vi "Text control 2 v5.9.vi"() -> ()   [LabVIEW 2016]
panel:
  in  "Tab Control":enum32{"Main", "Other parameters"}(tab)
  out "Line running":i32
  out "Total lines":i32
  out "Path":path=path "C:/users/rlp38/09Apr2009LTtesting/test2.txt"
  out "I vs Vg":cluster{"Y data in":dbl[], "X data in":dbl[]}[](graph)
  out "Is max":dbl format="%.2e"
  out "Id max":dbl format="%.2e"
  out "Ig max":dbl format="%.2e"
  out "Imax vs time":cluster{"Y data in":dbl[], "X data in":dbl[]}[](graph)
  out "Imin vs time":cluster{"Y data in":dbl[], "X data in":dbl[]}[](graph)
  out "I vs Vd":cluster{"Y data in":dbl[], "X data in":dbl[]}[](graph)
  in  "Script":string="#pulsedstressV d 0.03 20 0 0.5 0.0827 5\n#\n#itime m\n#gaterangemode a\n#drainrangemode a\n#pulsed on 0.05 0 0.02\n#transfer d -10 40 1 5 40 35\n#transfer d -10 40 1 5 40 35\n#transfer d -10 40 1 5 40 35\n#output d 0 40 20 0 40 1\n#\n#\n#sample 1 0.008 221 6 0.003\n#samplei 400e-6 200 6 0.002 0.1\n#vsu2pulse -10 4\n#\n#stressV 0.016 0.03 2e-4 0.1e-3 11\n#stressI 220e-7 0.08 15\n#transfer s -1 1 0.5 -0.005 0.005 0.005\n#output s 0 0 0 -0.008 0.008 0.002"
  out "Command running:":string
  out "Serial port data":string
  out "Elapsed Time":dbl caption="Elapsed Time (s)"
  in  "Units (label only)":u16(ring)=1 items=["Seconds", "Minutes", "Hours"]
  in  "Time Offset":dbl caption="Set Start Time (s)"
  in  "Reset":bool
  in  "Auto Reset":bool
  in  "integration time":u32(slide) max=2 step=1 scale=0.0..2.0
  out "Is on":dbl format="%.2e"
  out "Id on":dbl format="%.2e"
  out "Ig on":dbl format="%.2e"
  out "Ion vs time":cluster{"Y data in":dbl[], "X data in":dbl[]}[](graph)
  out "Ioff vs time":cluster{"Y data in":dbl[], "X data in":dbl[]}[](graph)
  out "Ig min":dbl format="%.2e"
  out "Id min":dbl format="%.2e"
  out "Is min":dbl format="%.2e"
  out "Is off":dbl format="%.2e"
  out "Id off":dbl format="%.2e"
  out "Ig off":dbl format="%.2e"
  in  "Integration time (long)":dbl=0.32 min=0.04 max=2.0 step=0.02 format="%.2f"
  in  "Integration time (short)":dbl=0.0019 min=8e-05 max=0.0019 step=8e-05 format="%^.0e"
  in  "Drain: Compliance":dbl=0.001 format="%.8f"
  in  "Gate: Compliance":dbl=0.001 format="%.8f"
  in  "Interrupt run":bool
  in  "Standby":T1
  in  "Full Reset":bool
  in  "SMU4":cluster{"on/off":bool, "Voltage":dbl} {"Voltage" min=-100.0 max=100.0 format="%.2f"}
  in  "Gate Range\nmode":u16(ring) items=["Auto", "Limited", "Fixed"]
  in  "Gate Range":u8(slide)=6 max=11 scale=0.0..11.0
  in  "Source/Drain\nRange mode":u16(ring) items=["Auto", "Limited", "Fixed"]
  in  "Source/Drain Range":u8(slide)=6 max=11 scale=0.0..11.0
  in  "Panel Controls":T2={"Emergency Stop"=refnum, "TransGraph Max"=1e-05, "Text/Graph (text=false)"=TRUE} {"TransGraph Max" format="%.2e"}
  in  "Panel Controls 2":T3={"Emergency Stop"=refnum, "TransGraph Max"=1e-05, "Text/Graph (text=false)"=TRUE, "TransGraph Min"=1e-11} {"TransGraph Min" format="%.2e"; "TransGraph Max" format="%.2e"}
  out "error out":errorcluster
  in  "Delay before read (ms)":u32=1000
  in  "byte count":u32=64
  in  "Serial End Mode for Reads":u16(ring)=2 items=["None", "LastBit", "TermChar"]
  in  "Timeout (ms)":u32=10000
  in  "Enable Termination\nChar (T)":bool=TRUE
  in  "Termination char\n(0xA = '\\n' = LF)\n(0xD = '\\r' = CR)":u8=13 format="%.0x"
  in  "flow control":u16(ring) items=["None"=0, "XON/XOFF"=1, "RTS/CTS"=2, "DTR/DSR"=4]
  in  "stop bits":u16(ring)=10 items=["1.0"=10, "1.5"=15, "2.0"=20]
  in  "parity":u16(ring) items=["None", "Odd", "Even", "Mark", "Space"]
  in  "data bits":u16=8 min=5 max=8 step=1
  in  "VISA resource name":refnum<visa-resource-name>="COM6"
  in  "baud rate":u32=9600
  out "Timings Indicator":T4
  in  "Timings (overwritten by the Front Panel)":T5={"integration time"=0, "Short/Long integration time"=0.00064, "hold time (sec)"=0.0, "delay time (sec)"=0.0, "Step Time (0 disables)"=0.0, "sweep method"=0, "Pulse period"=0.005, "Base voltage"=0.0, "Pulse width"=0.0005} {"Pulse width" min=0.0005 max=0.1 step=0.0001 format="%.4f"; "Base voltage" format="%^.4e"; "Pulse period" min=0.005 max=1.0 step=0.0001 format="%.4f"; "sweep method" items=["Continuous", "Pulsed"]; "Step Time (0 disables)" format="%.2f"; "delay time (sec)" format="%.4f"; "hold time (sec)" format="%.4f"; "Short/Long integration time" format="%^.0e"; "integration time" scale=0.0..2.0}
  in  "Gate":T6={"Gate Start"=0.0, "Gate Stop"=2.0, "Gate Step (linear only)"=1.0, "Gate Compliance"=0.0001, "Gate PComp"=0.0, "Range mode"=0, "Range"=6} {"Range" max=11 scale=0.0..11.0; "Range mode" items=["Auto", "Limited", "Fixed"]; "Gate PComp" format="%^.2e"; "Gate Compliance" format="%^.2e"; "Gate Step (linear only)" format="%^.4e"; "Gate Stop" format="%^.4e"; "Gate Start" format="%^.4e"}
  in  "Drain 2":T7={"Drain Start"=0.0, "Drain Stop"=2.0, "Drain Compliance"=0.0001, "Drain Step"=1.0, "Drain PComp"=0.0, "Range mode"=0, "Range"=6} {"Range" max=11 scale=0.0..11.0; "Range mode" items=["Auto", "Limited", "Fixed"]; "Drain PComp" format="%^.2e"; "Drain Step" format="%^.4e"; "Drain Compliance" format="%^.2e"; "Drain Stop" format="%^.4e"; "Drain Start" format="%^.4e"}
  # "Time"
  # "Syntax:\nitime [s|m|l] time(sec): [s|m|l] determines the integration time setting (small|medium|long) and time sets the value.\nNOTE: The value of the integration time has to be within the range allowed by its category (s|m|l), otherwise, the closest value will be used. (e.g. if the category is set to short but the time value is very long, the actual value used will be the maximum short integration time.\nIntegration times:\n    Short: Default: 640 us. Range: 8E-5 - 1.92E-3 seconds.\n    Medium: Fixed at 1 NPL cycle (0.02 seconds).\n    Long: Default: 16 NPL cycles (0.32 seconds). Range: 2-100 NPL cycles (0.04 seconds - 2 seconds).\ngaterangemode [a|l|f]\ndrainrangemode [a|l|f]\npulsed [on|off] PulsePeriod(sec) PulseBaseVoltage PulseONWidth(sec)\nstandby [on l off]\nwait NumMilliseconds\nwait-min NumMinutes\n# texthere = comment\ntransfer [s|d] VgStart VgStop VgStep VdStart VdStop VdStep\noutput [s|d] VgStart VgStop VgStep VdStart VdStop VdStep\nsample Vg Vd NumSamples Time(s) SampleInterval(s)\nsamplei Idg NumSamples Time(s) SampleInterval(s) VDGcompliance\n100 samples is approximately 13 seconds with medium integration\n# if in doubt use SampleInterval(s) = 0.004\nstressV VG VD IGcompliance IDcompliance Duration(sec)\nstressI IDG VDGcompliance Duration(sec)\nvsu2pulse Bias Duration(s)\npulsedstressV [s|d] VEstop VgON VgOFF Period(s) PulseONwidth(s) Vd\nsample-fpp Vg Vd NumSamples Time\nresample-fpp Vg Vd\ntransfer-fpp [s|d] VgStart VgStop VgStep VdStart VdStop VdStep\noutput-fpp [s|d] VgStart VgStop VgStep VdStart VdStop VdStep\nserial SerialPortCommand"
  # "1\n2\n3\n4\n5\n6\n7\n8\n9\n10\n11\n12\n13\n14\n15\n16\n17\n18\n19\n20"
  # "Serial port settings"
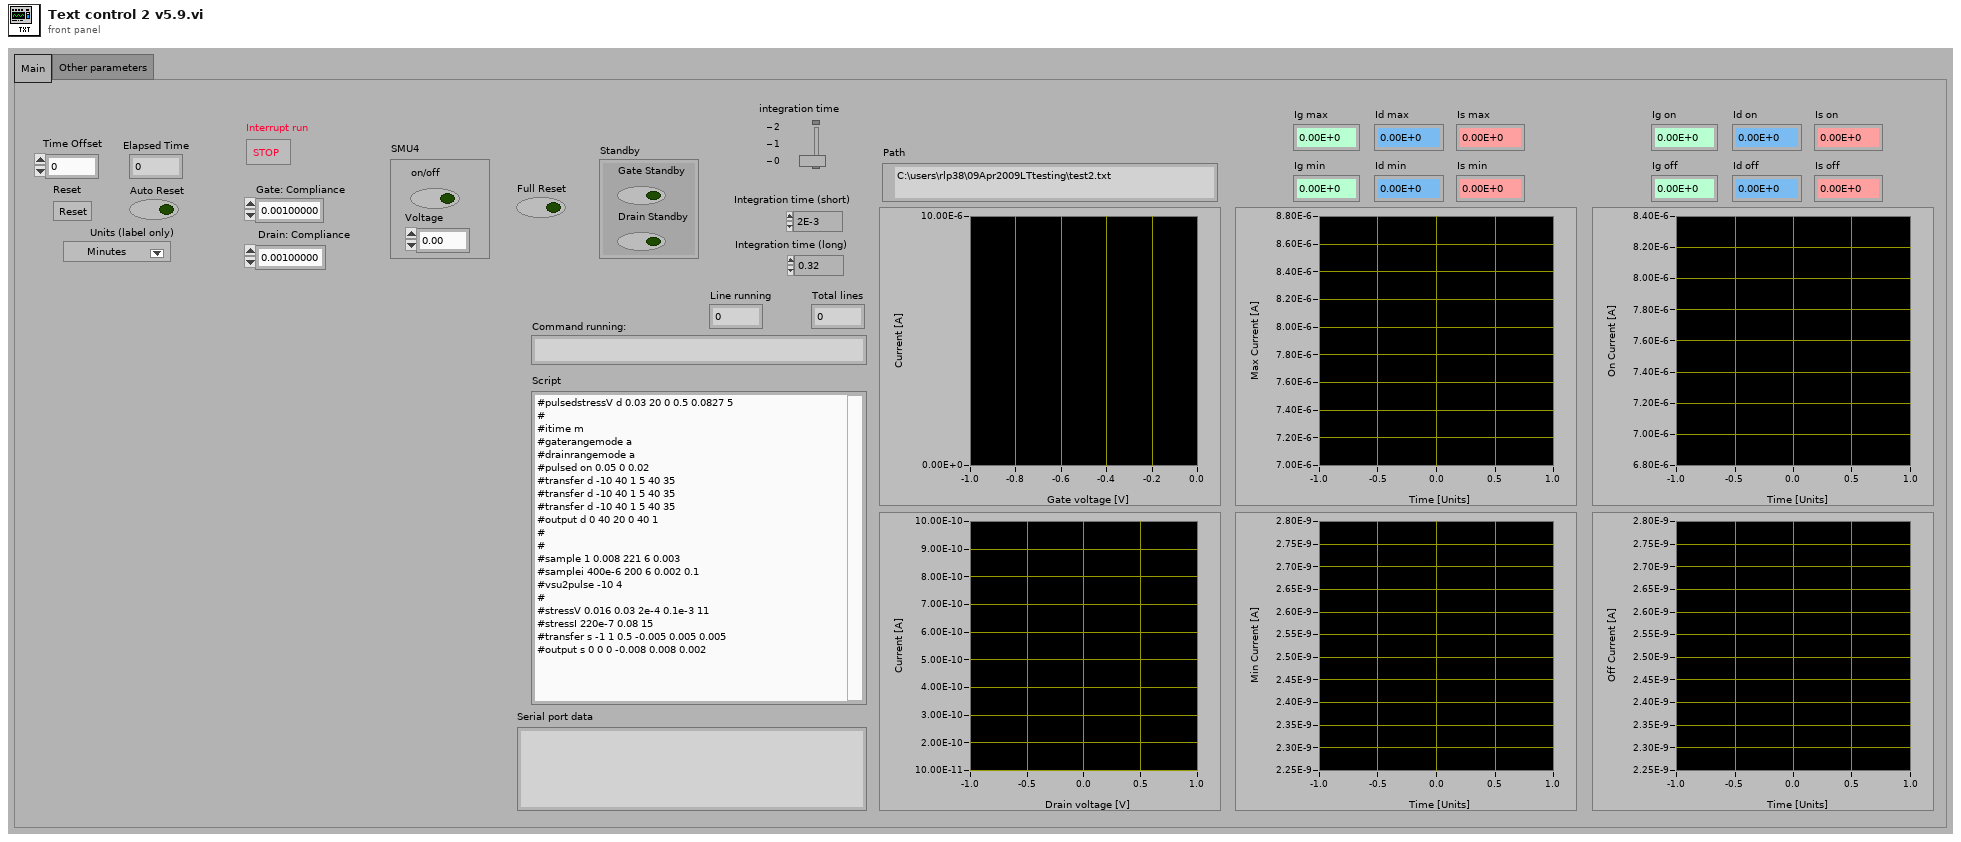
[diagram p1: front panel]
types:
  T1 = cluster{"Gate Standby":bool, "Drain Standby":bool}
  T2 = cluster{"Emergency Stop":refnum<vi>, "TransGraph Max":dbl, "Text/Graph (text=false)":bool}
  T3 = cluster{"Emergency Stop":refnum<vi>, "TransGraph Max":dbl, "Text/Graph (text=false)":bool, "TransGraph Min":dbl}
  T4 = cluster{"integration time (0:s, 1:m, 2:l)":u32, "Short/Long integration time":dbl, "hold time (sec)":dbl, "delay time (sec)":dbl, "Step Time (0 disables)":dbl, "sweep method":u16, "Pulse period":dbl, "Base voltage":dbl, "Pulse width":dbl}
  T5 = cluster{"integration time":u32, "Short/Long integration time":dbl, "hold time (sec)":dbl, "delay time (sec)":dbl, "Step Time (0 disables)":dbl, "sweep method":u16, "Pulse period":dbl, "Base voltage":dbl, "Pulse width":dbl}
  T6 = cluster{"Gate Start":dbl, "Gate Stop":dbl, "Gate Step (linear only)":dbl, "Gate Compliance":dbl, "Gate PComp":dbl, "Range mode":u16, "Range":u8}
  T7 = cluster{"Drain Start":dbl, "Drain Stop":dbl, "Drain Compliance":dbl, "Drain Step":dbl, "Drain PComp":dbl, "Range mode":u16, "Range":u8}
  T8 = enum16{"open", "replace", "create", "open or create", "replace or create", "replace or create with confirmation"}
  T9 = cluster{"V2 Start":dbl, "V2 Step":dbl, "Number of points":i32}
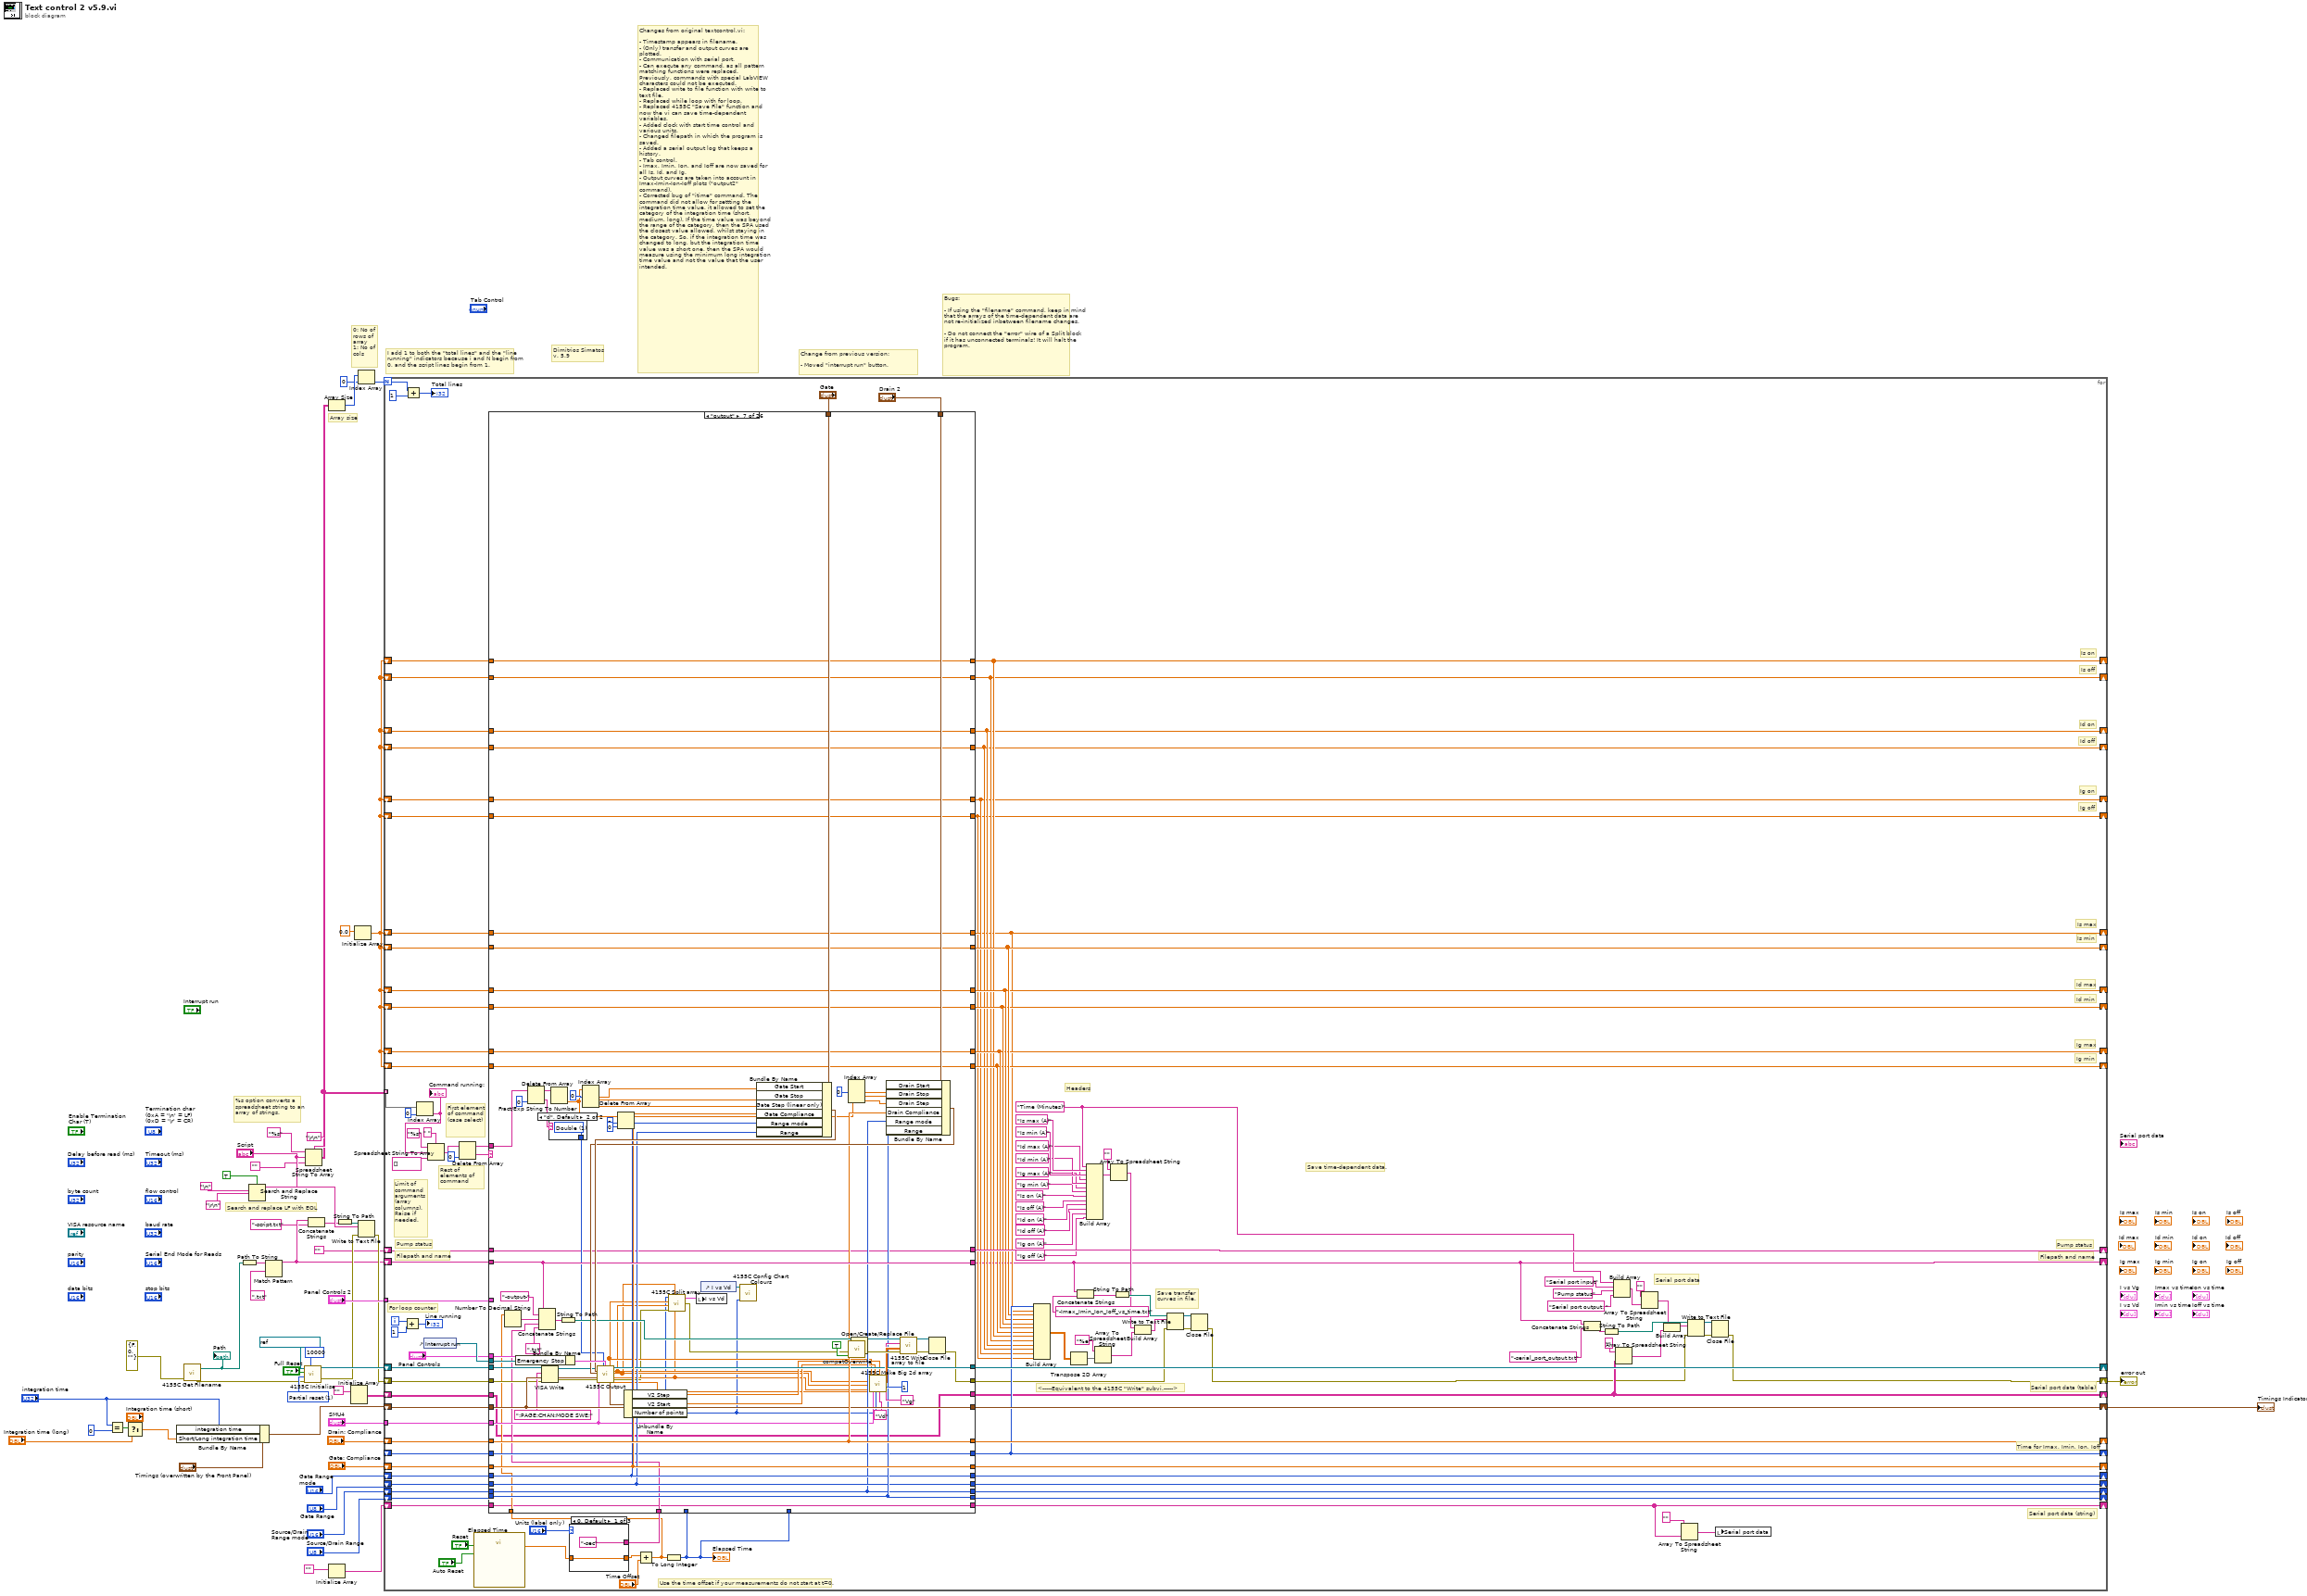
[diagram p0: block diagram]
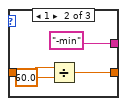
[diagram p2: hidden frame]
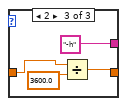
[diagram p3: hidden frame]
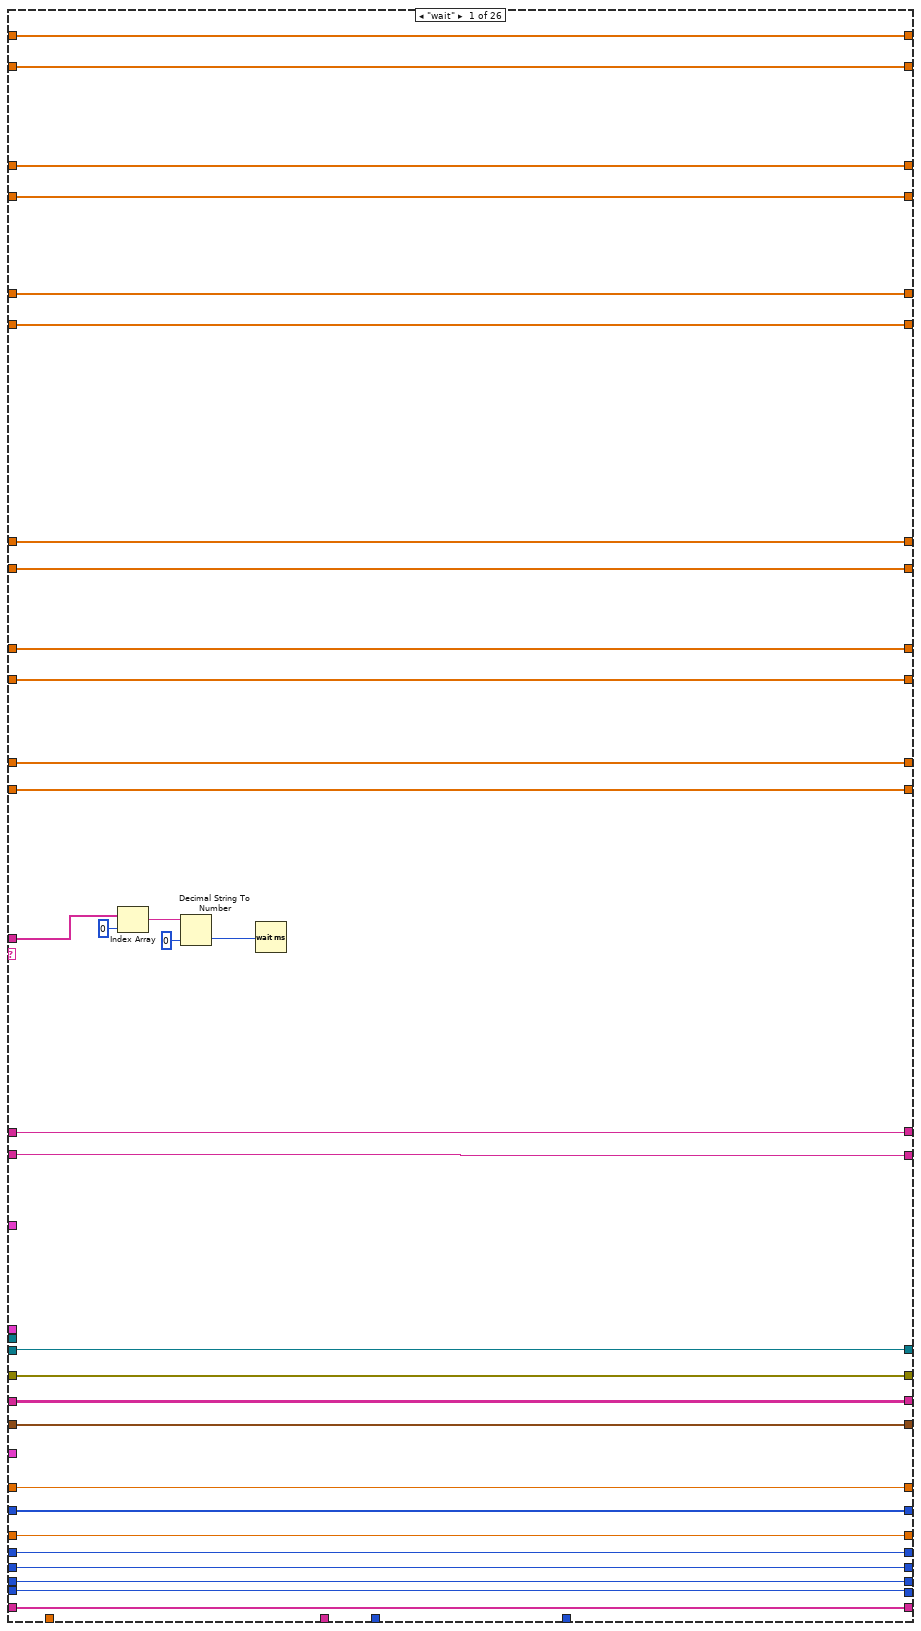
[diagram p4: hidden frame]
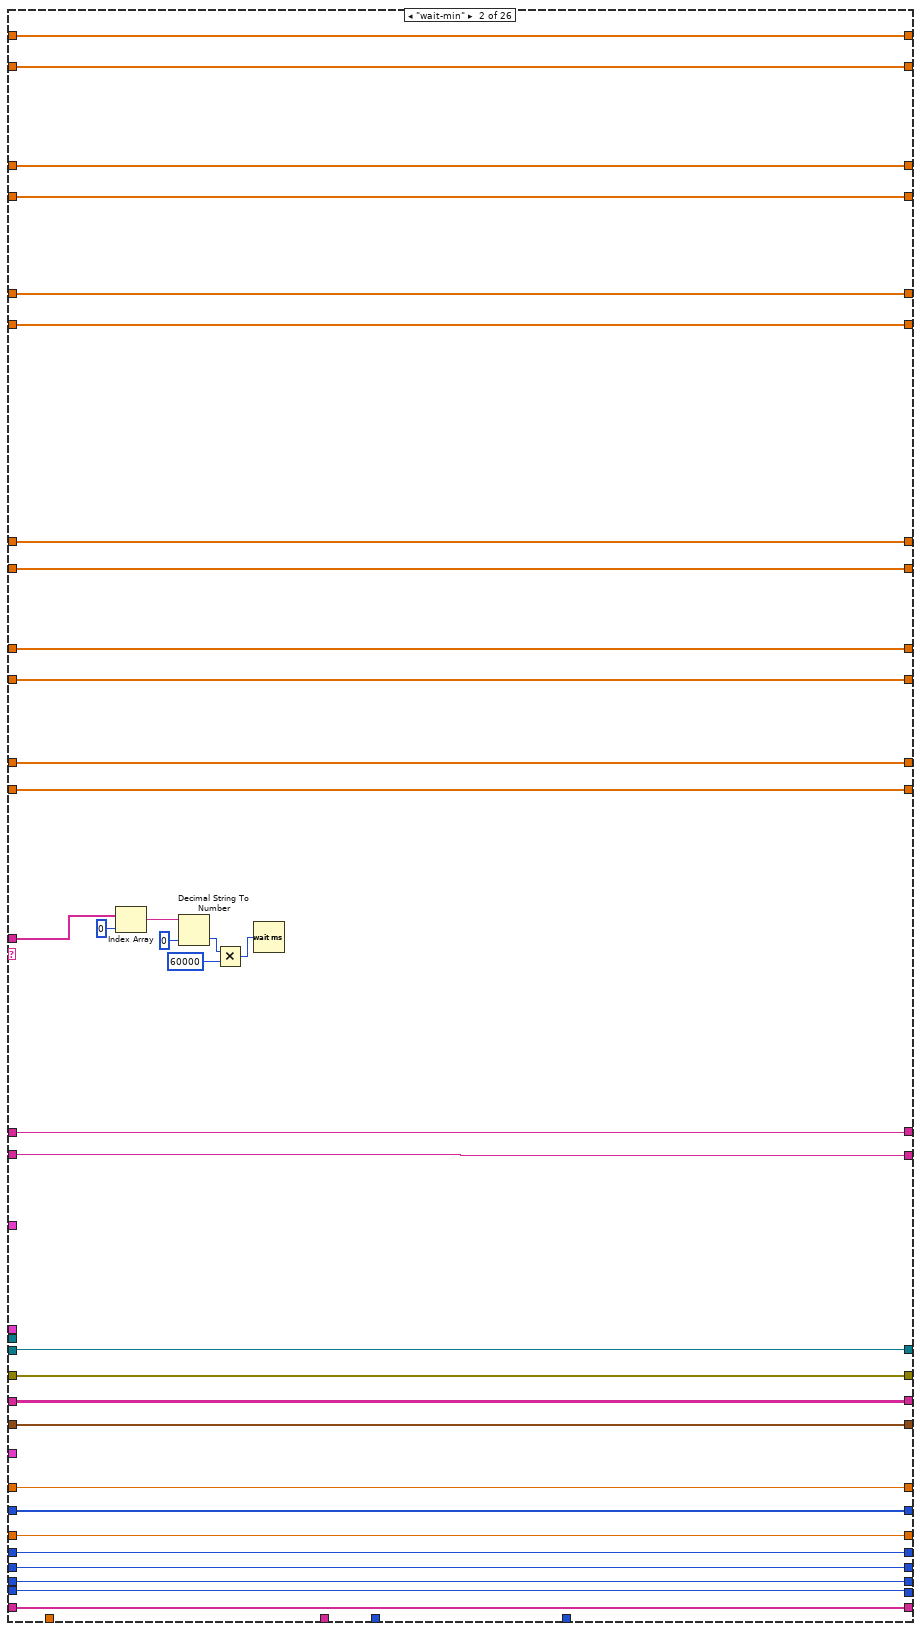
[diagram p5: hidden frame]
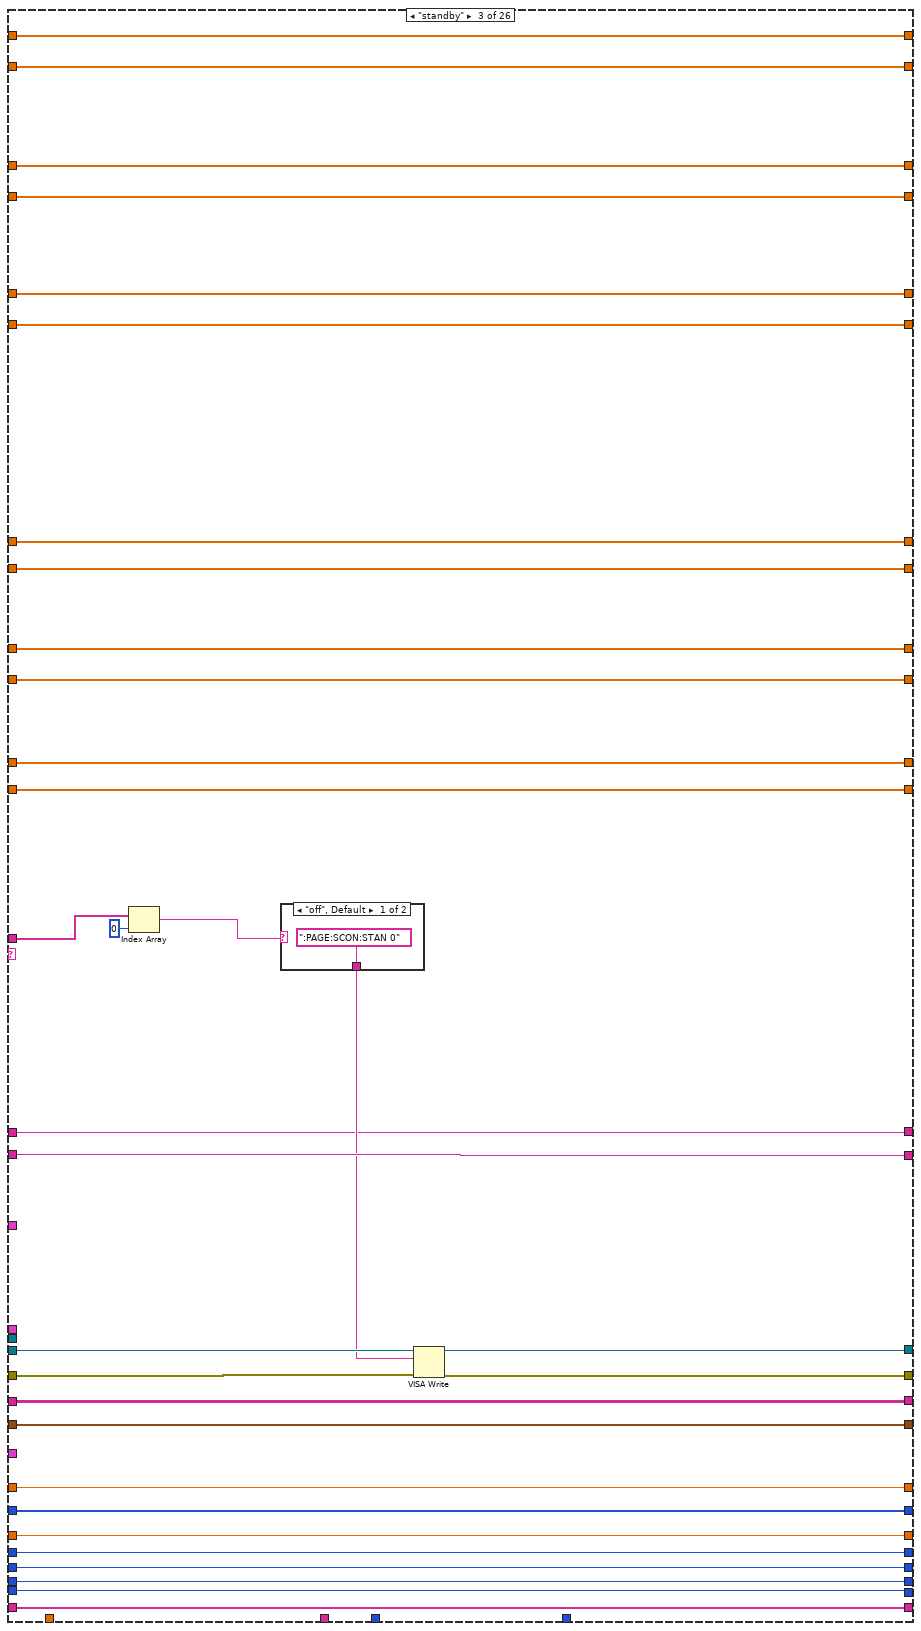
[diagram p6: hidden frame]
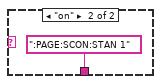
[diagram p7: hidden frame]
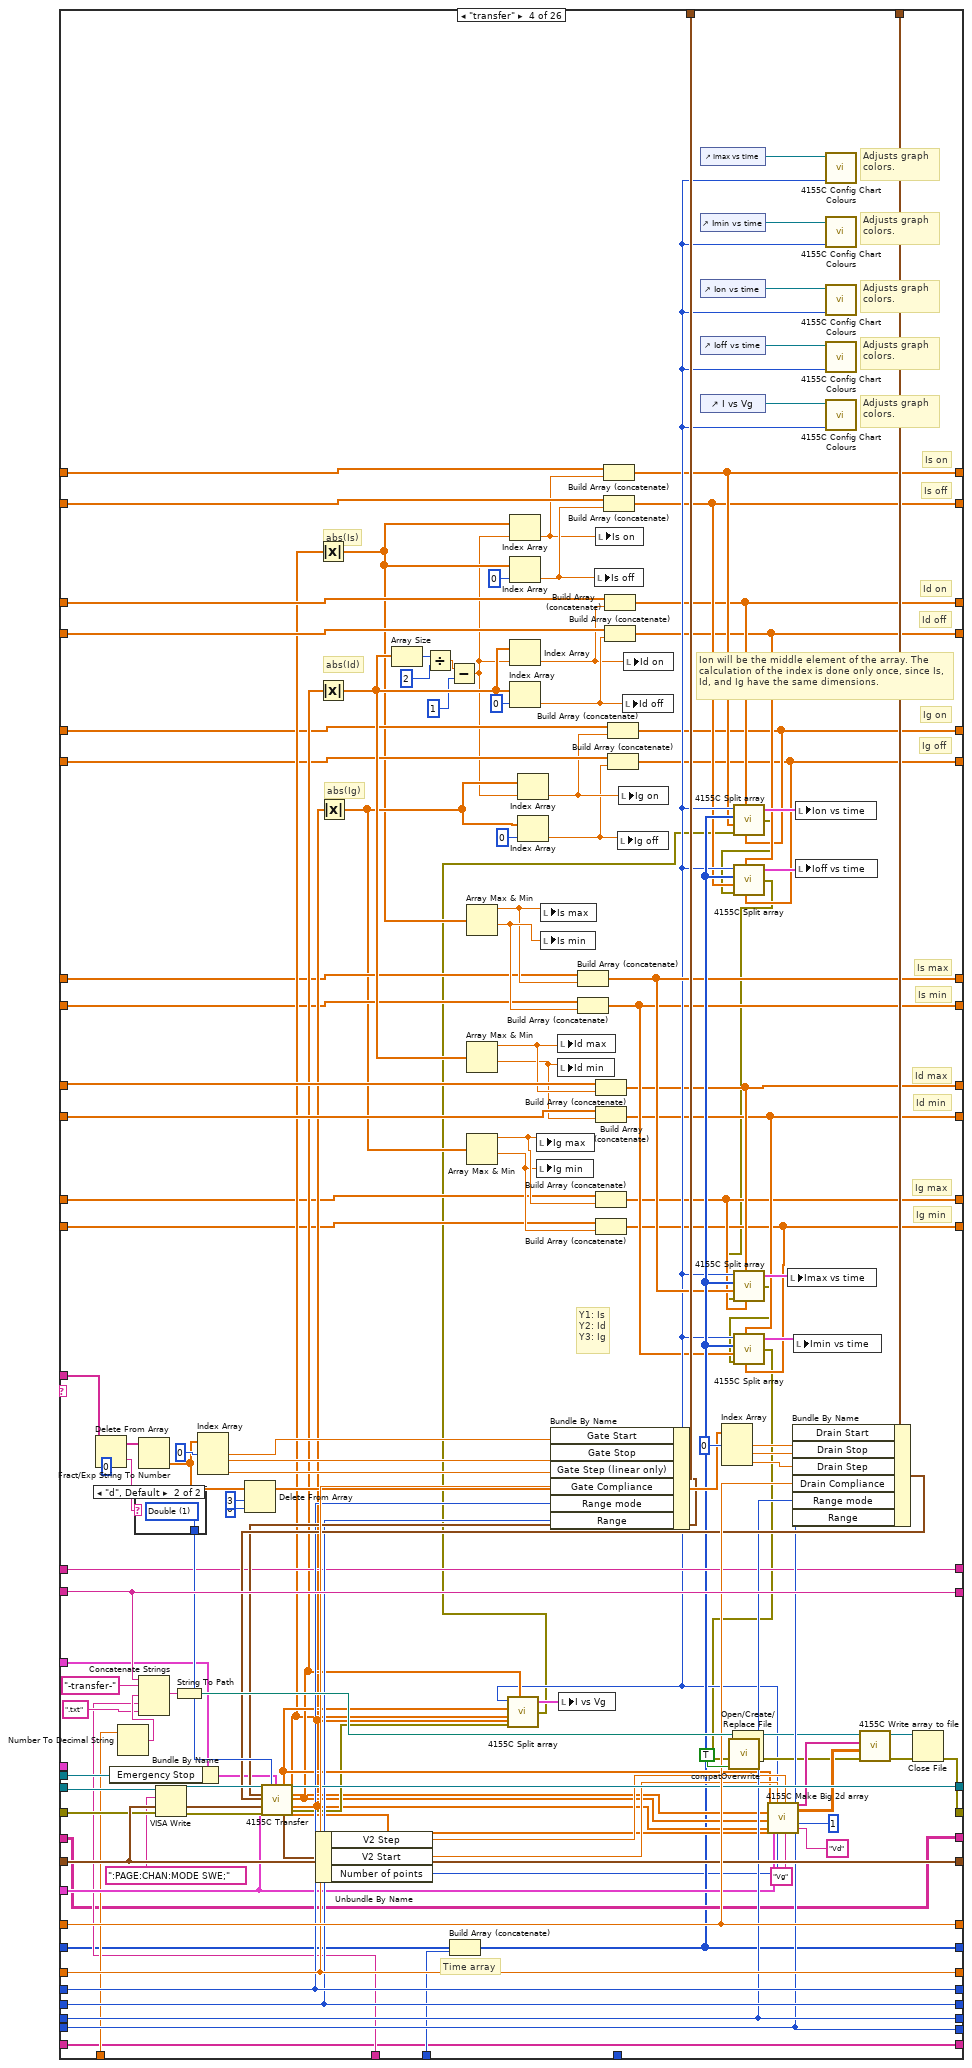
[diagram p8: hidden frame]
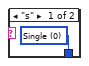
[diagram p9: hidden frame]
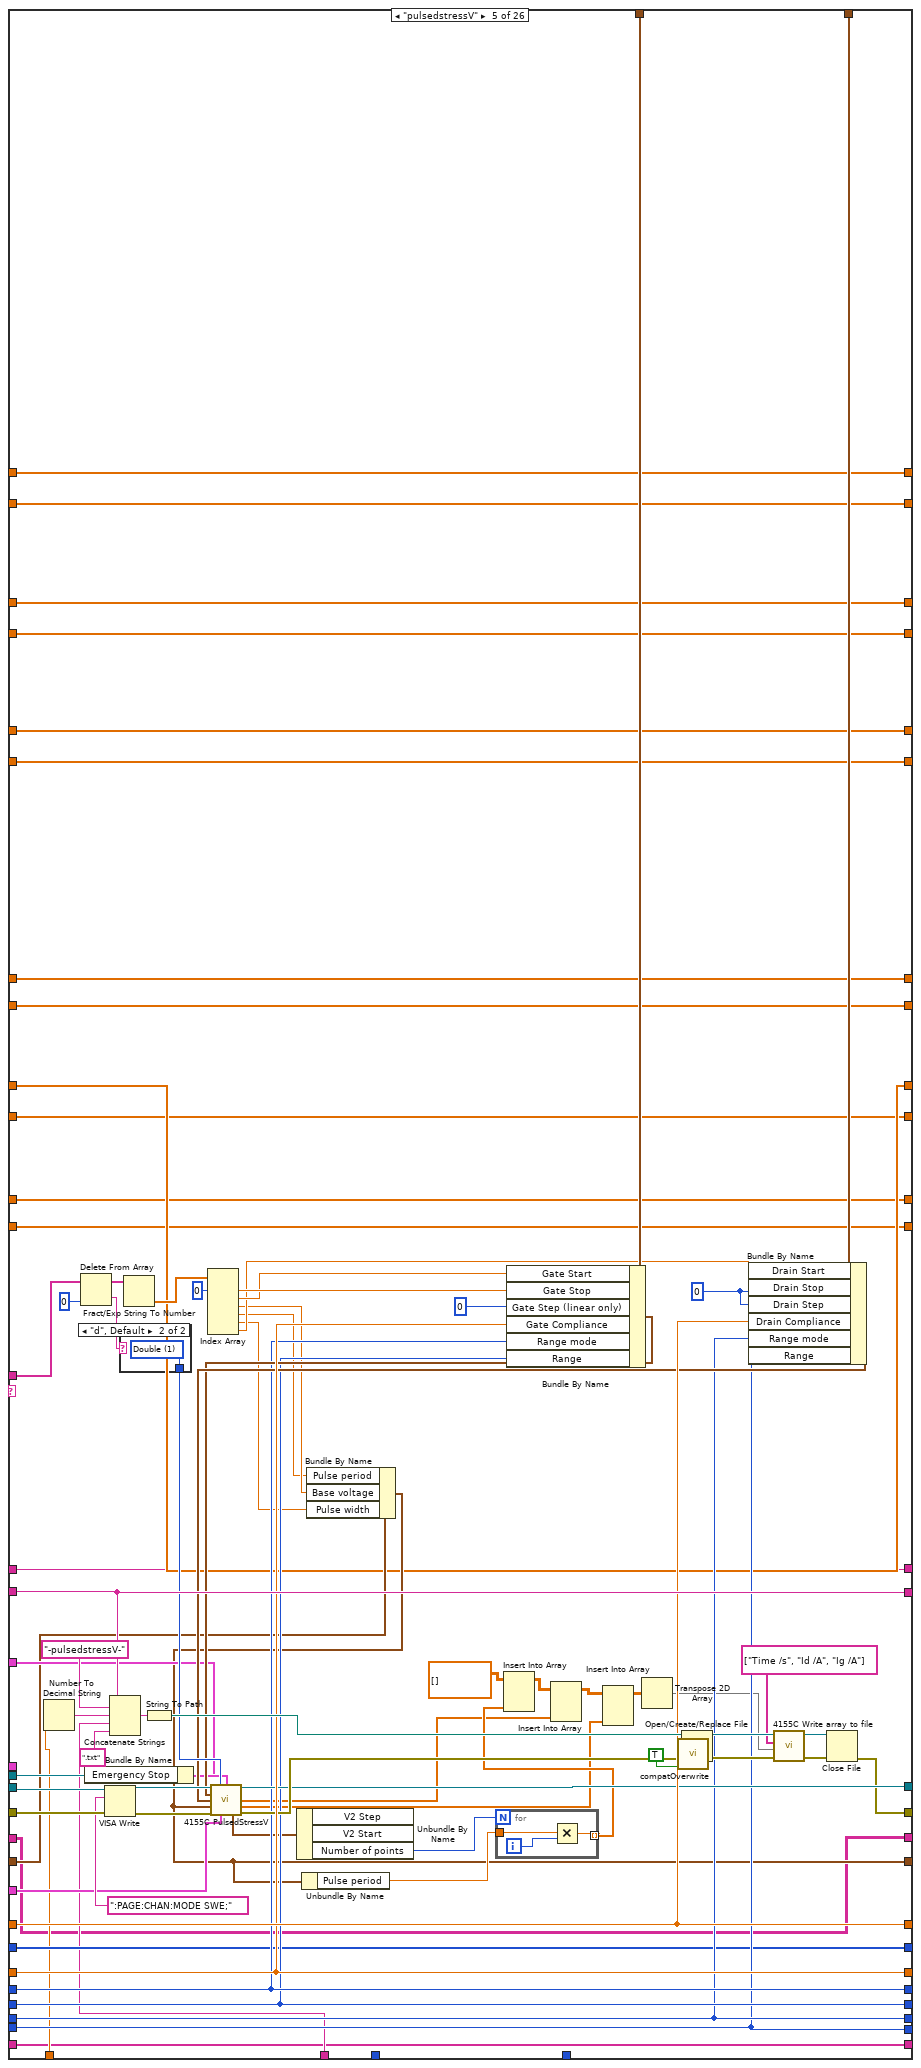
[diagram p10: hidden frame]
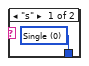
[diagram p11: hidden frame]
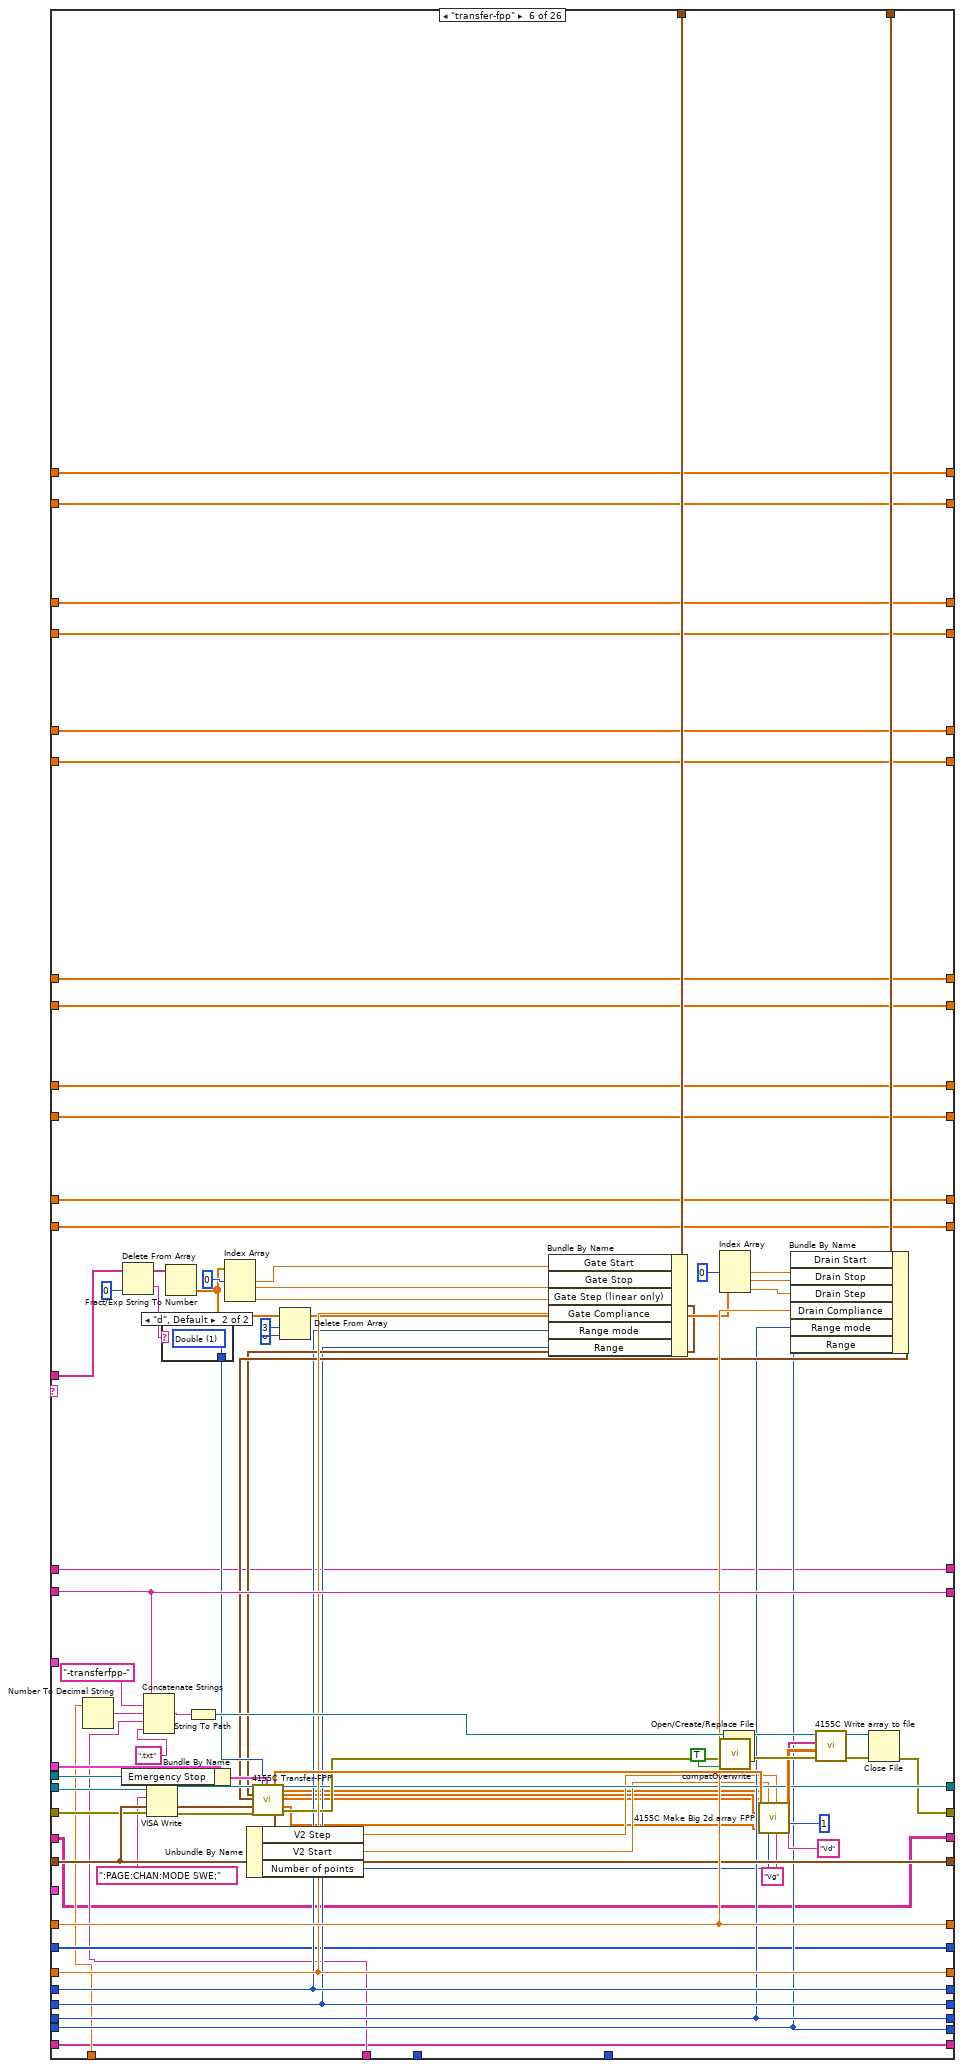
[diagram p12: hidden frame]
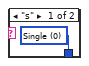
[diagram p13: hidden frame]
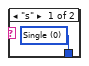
[diagram p14: hidden frame]
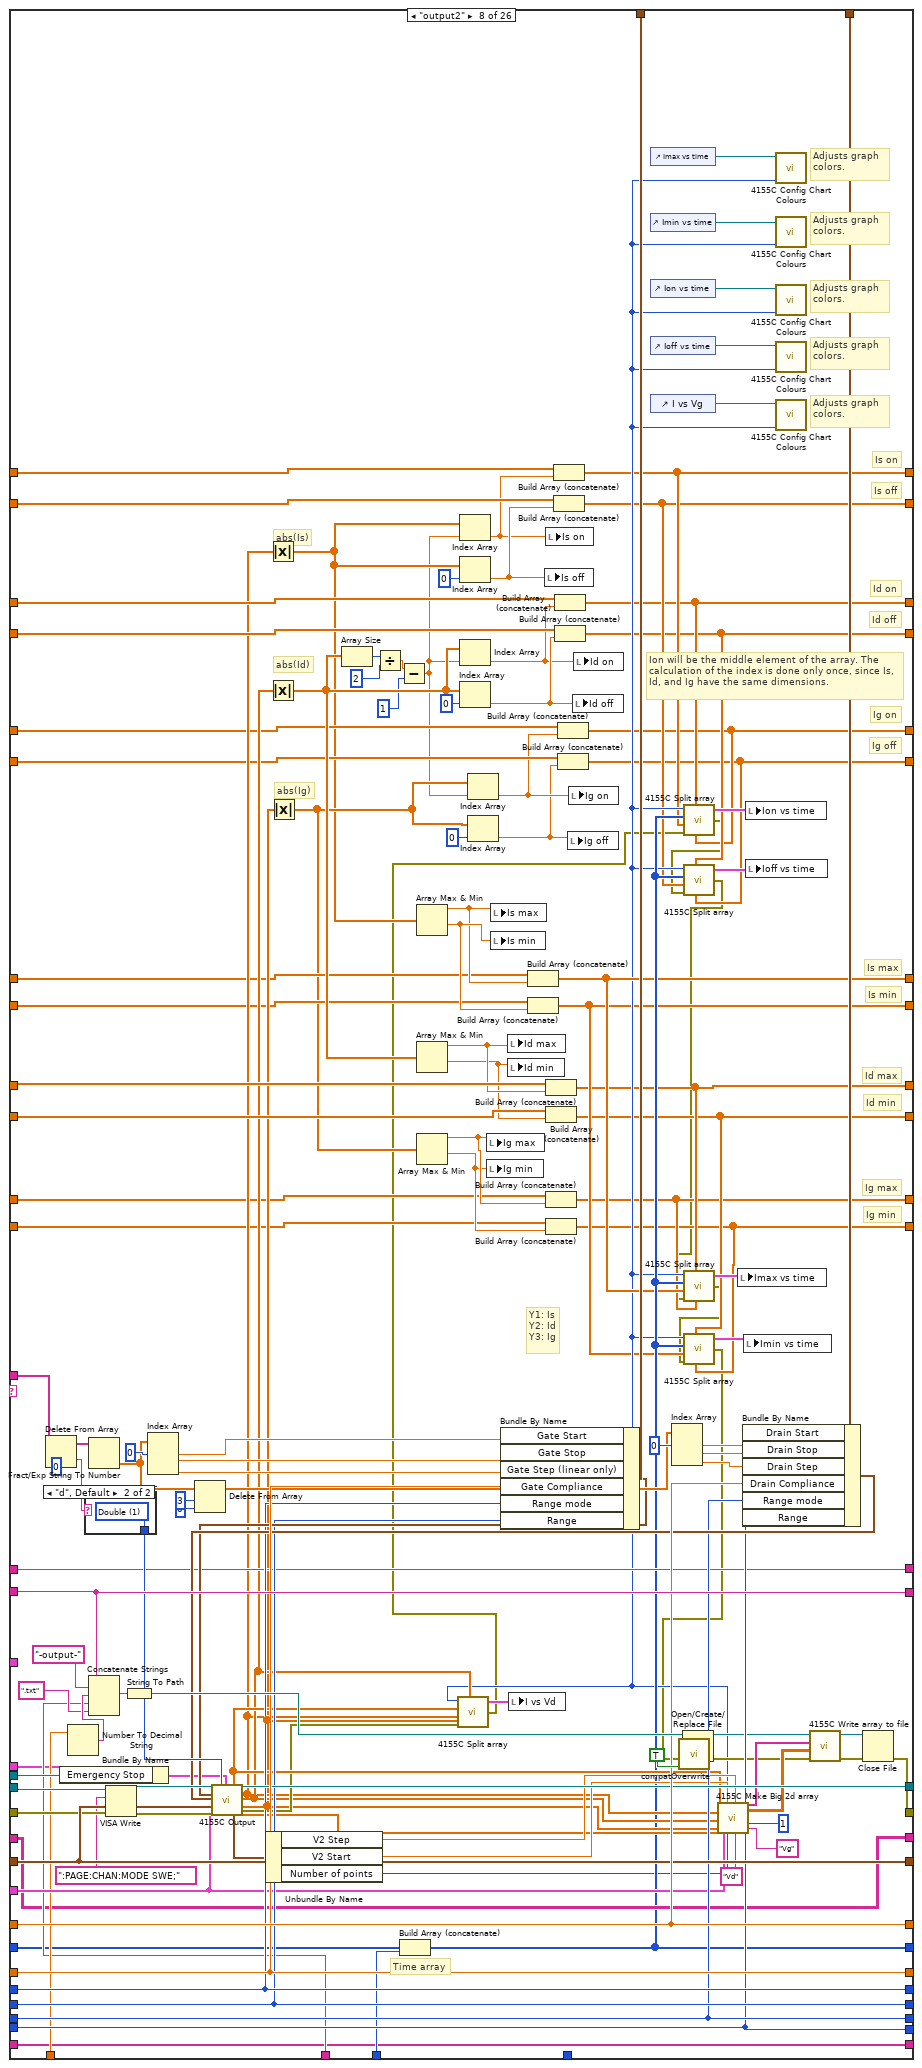
[diagram p15: hidden frame]
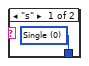
[diagram p16: hidden frame]
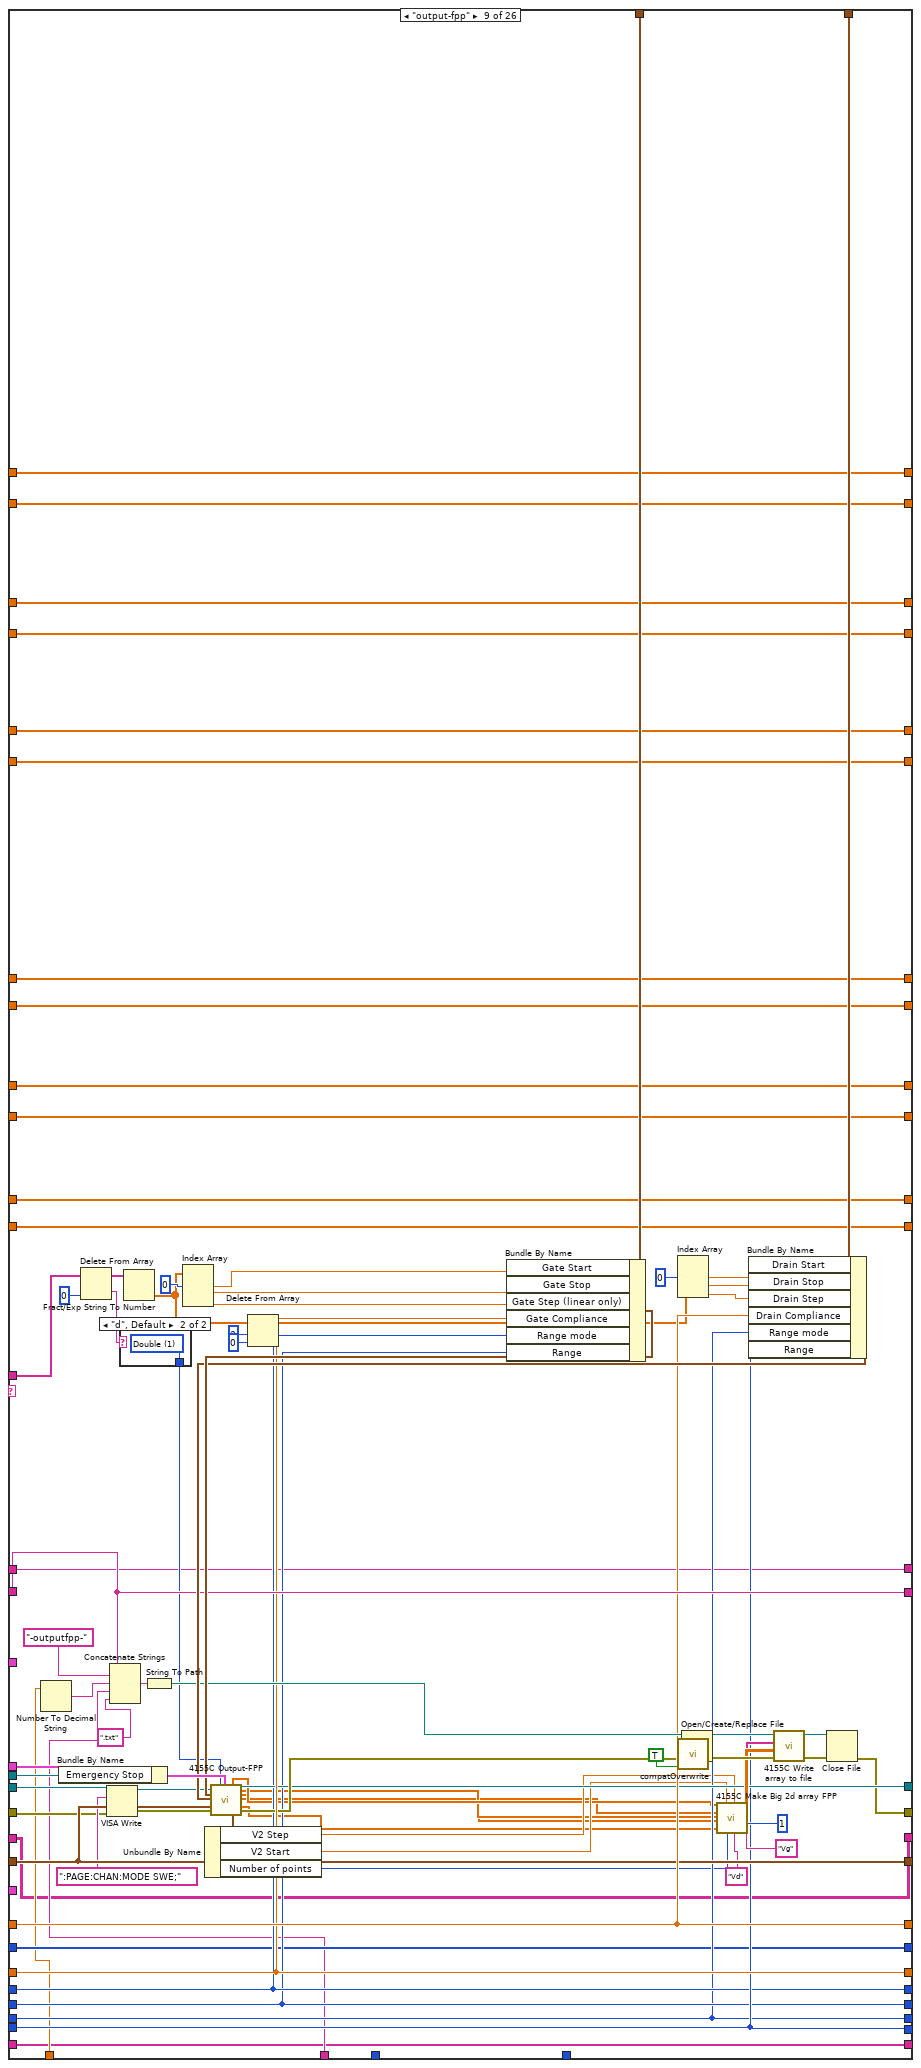
[diagram p17: hidden frame]
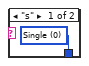
[diagram p18: hidden frame]
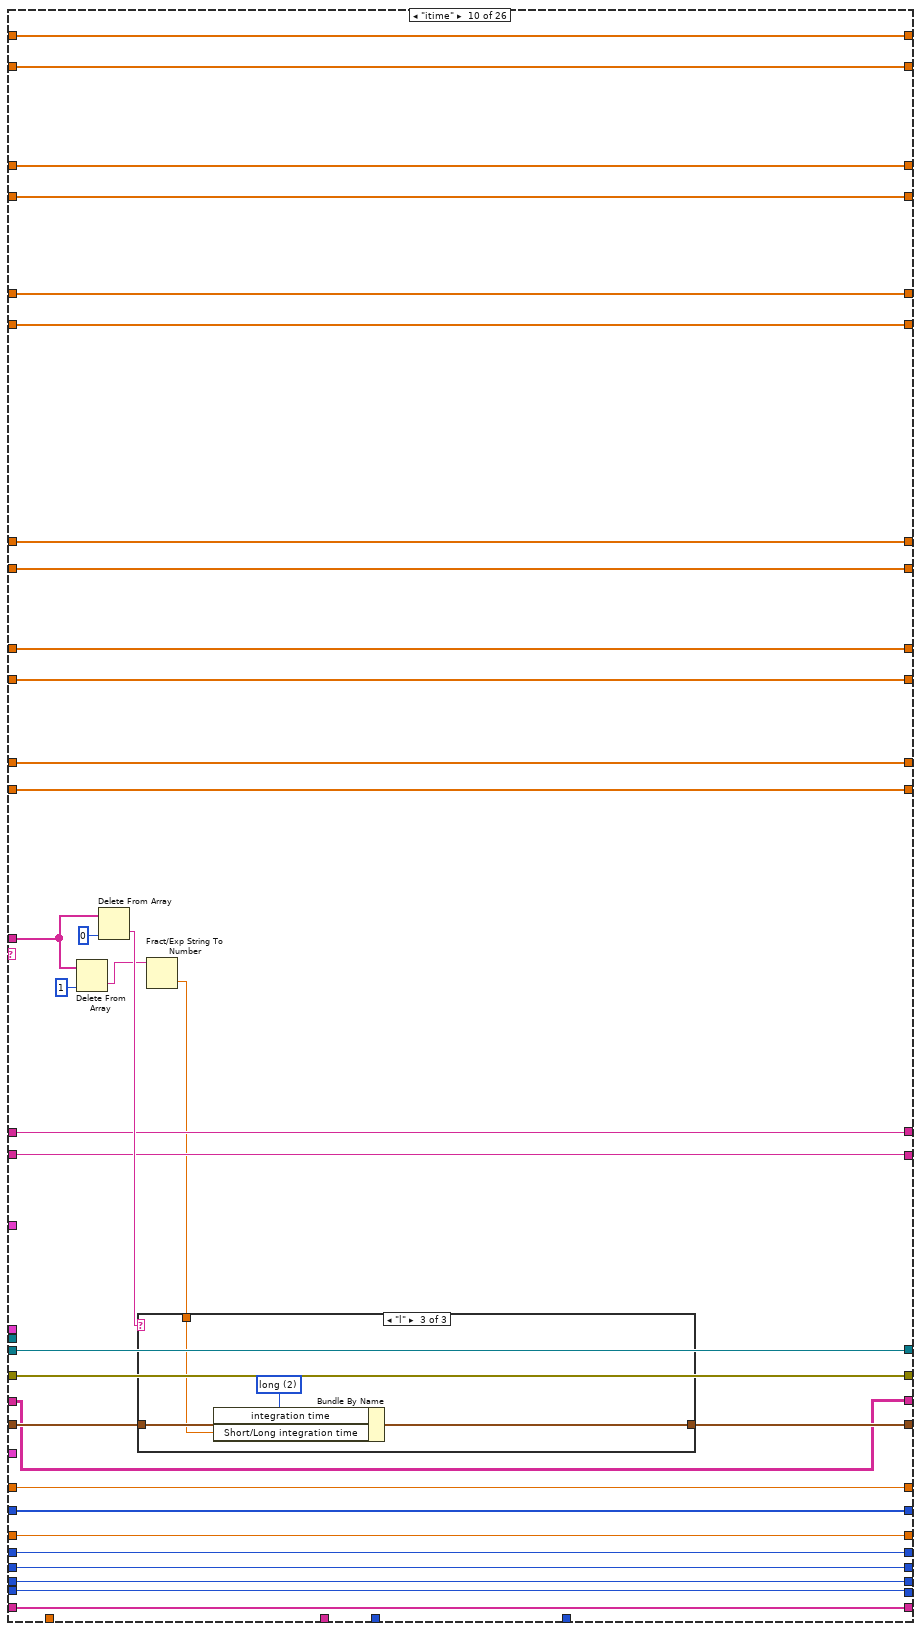
[diagram p19: hidden frame]
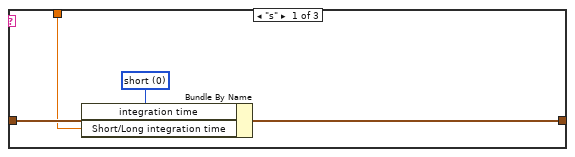
[diagram p20: hidden frame]
diagram:
  w48 = u16 1 items=["Reset All", "Partial reset"] ("Type of reset")
  # "Change from previous version:\n\n- Moved \"interrupt run\" button."
  # "I add 1 to both the \"total lines\" and the \"line running\" indicators because i and N begin from 0, and the script lines begin from 1."
  # "Bugs:\n\n- If using the \"filename\" command, keep in mind that the arrays of the time-dependent data are not re-initialized inbetween filename changes. \n\n- Do not connect the \"error\" wire of a Split block if it has unconnected terminals! It will halt the program."
  # "Array size"
  # "%s option converts a spreadsheet string to an array of strings."
  # "0: No of rows of array\n1: No of cols"
  # "Dimitrios Simatos\nv. 5.9"
  # "Changes from original textcontrol.vi:\n\n- Timestamp appears in filename.\n- (Only) transfer and output curves are plotted.\n- Communication with serial port.\n- Can execute any command, as all pattern matching functions were replaced. Previously, commands with special LabVIEW characters could not be executed.\n- Replaced write to file function with write to text file.\n- Replaced while loop with for loop.\n- Replaced 4155C \"Save File\" function and now the vi can save time-dependent variables.\n- Added clock with start time control and various units.\n- Changed filepath in which the program is saved.\n- Added a serial output log that keeps a history.\n- Tab control.\n- Imax, Imin, Ion, and Ioff are now saved for all Is, Id, and Ig.\n- Output curves are taken into account in Imax-Imin-Ion-Ioff plots (\"output2\" command).\n- Corrected bug of \"itime\" command. The command did not allow for settting the integration time value, it allowed to set the category of the integration time (short, medium, long). If the time value was beyond the range of the category, then the SPA used the closest value allowed, whilst staying in the category. So, if the integration time was changed to long, but the integration time value was a short one, then the SPA would measure using the minimum long integration time value and not the value that the user intended."
  # "Search and replace LF with EOL"
  n1 = Equal?(x="integration time", y=u32 0) -> (x = y?=w49:bool)
  n2 = Select(t="Integration time (short)", s=w49, f="Integration time (long)") -> (s? t:f=w4:dbl)
  n3 = Bundle By Name(cluster="Timings (overwritten by the Front Panel)", "integration time"="integration time", "Short/Long integration time"=w4) -> (w41:T5)
  n4 = call "4155C Get Filename.vi"("error in (no error)"=errorcluster {"status"=FALSE, "code"=0, "source"=""}) -> ("error out"=w43:errorcluster, "path"=w18:path)  [unwired: 2 in, 1 out]
  "Path" <- w18
  n5 = Path To String(path=w18) -> (string=w19:string)
  n6 = Search and Replace String(replace all?=TRUE ("replace all? (F)"), input string="Script", search string="\n", replace string="\r\n") -> (result string=w31:string)  [unwired: 4 in, 3 out]
  n7 = Match Pattern(string=w19, regular expression=".txt") -> (before substring=w2:string)  [unwired: 1 in, 3 out]
  n8 = call "4155C Initialise.vi"("VISA resource name in"=refnum<visa-resource-name> "GPIB0::14::INSTR", "Reset"="Full Reset", "Type of reset"=w48, "error in (no error)"=w43, "VISA Timeout Value"=u32 10000) -> ("VISA Resource Name out"=w42:refnum<visa-resource-name>, "error out"=w14:errorcluster)
  n9 = Spreadsheet String To Array(delimiter (Tab)="\r\n", format string="%s", spreadsheet string="Script", array type (2D Dbl)="") -> (array=w22:string[][])
  n10 = Concatenate Strings(w2, "-script.txt" ("string")) -> (w3:string)
  n11 = Array Size(array=w22) -> (size(s)=w26:i32[])
  n12 = Initialize Array("") -> (w9:string[])  [unwired: 1 in]
  n13 = String To Path(string=w3) -> (path=w15:path)
  n14 = Initialize Array("") -> (w7:string[][])  [unwired: 2 in]
  n15 = Initialize Array(0.0 ("element")) -> (w11:dbl[])  [unwired: 1 in]
  n16 = Index Array(array=w26, index=0) -> (element=w24:i32)
  n17 = Write to Text File(file (use dialog)=w15, text=w31, error in=w14) -> (error out=w13:errorcluster)  [unwired: 1 in, 2 out]
  n18 = for {
    N: w24 -> [w122]
    tunnel: "SMU4" -> [w158]
    shift-left: "Source/Drain Range" -> [w163]
    shift-right: [w159] -> _
    shift-left: "Source/Drain\nRange mode" -> [w164]
    shift-right: [w160] -> _
    shift-left: "Gate Range" -> [w165]
    shift-right: [w161] -> _
    shift-left: "Gate Range\nmode" -> [w166]
    shift-right: [w162] -> _
    shift-left: "Gate: Compliance" -> [w175]
    shift-right: [w171] -> _
    shift-left: "Drain: Compliance" -> [w176]
    shift-right: [w172] -> _
    shift-left: w41 -> [w177]
    shift-right: [w173] -> w5
    shift-left: w13 -> [w178]
    shift-right: [w54] -> w17
    shift-left: w42 -> [w179]
    shift-right: [w174] -> _
    shift-left: w2 -> [w180]
    shift-right: [w57] -> _
    tunnel: "Panel Controls 2" -> [w157]
    shift-right: [w69] -> _
    shift-left: w11 -> [w156]
    shift-right: [w107] -> _
    shift-left: _ -> [w152]
    tunnel: w22 -> [w151] mode=indexing
    shift-right: [w68] -> _
    shift-left: w11 -> [w128]
    shift-right: [w101] -> _
    shift-left: w9 -> [w114]
    shift-right: [w109] -> _
    shift-left: "" -> [w108]
    shift-right: [w102] -> _
    shift-left: w7 -> [w104]
    shift-right: [w62] -> _
    shift-left: w11 -> [w90]
    shift-right: [w63] -> _
    shift-left: w11 -> [w89]
    shift-right: [w67] -> _
    shift-left: w11 -> [w78]
    shift-right: [w66] -> _
    shift-left: w11 -> [w77]
    shift-right: [w60] -> _
    shift-left: w11 -> [w76]
    shift-right: [w70] -> _
    shift-left: w11 -> [w75]
    shift-right: [w61] -> _
    shift-left: w11 -> [w74]
    shift-right: [w59] -> _
    shift-left: w11 -> [w73]
    shift-right: [w65] -> _
    shift-left: w11 -> [w72]
    shift-right: [w64] -> _
    shift-left: w11 -> [w71]
    i -> [w117]
    w92 = "Time (Minutes)" ("element")
    # "Is off"
    # "Is on"
    # "Ig off"
    # "Ig on"
    # "Is min"
    # "Is max"
    # "Ig min"
    # "Ig max"
    # "Id min"
    # "Id max"
    # "Id off"
    # "Id on"
    # "Pump status"
    # "Filepath and name"
    # "Pump status"
    # "Limit of command arguments (array columns). Raise if needed."
    # "Serial port data (string)"
    # "Serial port data (table)"
    # "Serial port data"
    # "For loop counter"
    # "<-----Equivalent to the 4155C \"Write\" subvi.----->"
    # "Headers"
    # "Save transfer curves in file."
    # "Filepath and name"
    # "Save time-dependent data."
    # "Use the time offset if your measurements do not start at t=0."
    # "Time for Imax, Imin, Ion, Ioff"
    # "Rest of elements of command"
    # "First element of command\n(case select)"
    n19 = Add(x=w117, y=1) -> (x+y=→"Line running":i32)
    n20 = Add(x=w122, y=1) -> (x+y=→"Total lines":i32)
    n21 = Index Array(array=w151, index=0 ("line index")) -> (element=w146:string)
    "Command running:" <- w146
    n22 = control-ref of="Interrupt run"() -> (w170:refnum<vi>)
    n23 = Spreadsheet String To Array(delimiter (Tab)=" ", format string="%s", spreadsheet string=w146, array type (2D Dbl)=string[] []) -> (array=w144:string[])
    n24 = Delete From Array(array=w144, index=0) -> (deleted portion=w91:string, array with subset deleted=w143:string[])  [unwired: 1 in]
    n25 = call "Elapsed Time"("Reset"="Reset", "Auto Reset"="Auto Reset") -> ("Elapsed Time (s)"=w153:dbl)  [unwired: 10 in, 7 out]
    n26 = case shown="0, Default" "Units (label only)" {
      tunnel: ["-sec" "-min" "-h"] -> w154
      tunnel: [w181 w185 w188] -> w124
      tunnel: w153 -> [w181 w184 w189]
      frame 0, Default {
      }
      frame 1 {
        n27 = Divide(x=w184, y=60.0) -> (x/y=w185:dbl)
      }
      frame 2 {
        n28 = Divide(x=w189, y=3600.0) -> (x/y=w188:dbl)
      }
    }
    n29 = Add(x=w124, y="Time Offset") -> (x+y=w123:dbl)
    n30 = To Long Integer(number=w123) -> (32bit integer=w106:i32)
    "Elapsed Time" <- w106
    n31 = case shown="\"output\"" w91 {
      tunnel: w143 -> [w221 w254 w286 w414 w437 w574 w664 w812 w885 w912 w982 w1023 w1062 w1097 w1125 _ _ w1271 w1346 _ w1439 w1497 w1553 w1637 w1713 w1747]
      tunnel: w180 -> [w216 w250 w284 w421 w498 w582 w671 w819 w893 w930 w971 w1015 w1055 w1091 w1118 w1151 w1207 w1249 w1328 w1373 w1426 w1484 w1541 w1631 w1709 w1749]
      tunnel: w179 -> [w215 w249 w275 w392 w483 w551 w640 w790 w861 w931 w972 w1016 w1056 w1092 w1119 w1156 w1209 w1277 w1352 w1377 w1445 w1503 w1559 w1643 w1667 w1753]
      tunnel: w178 -> [w214 w248 w274 w391 w482 w550 w637 w789 w858 w932 w973 w1017 w1057 w1093 w1120 w1155 w1180 w1276 w1351 w1376 w1444 w1502 w1558 w1642 w1666 w1752]
      tunnel: w177 -> [w213 w247 w283 w417 w458 w578 w667 w815 w889 w940 w981 w1014 w1054 w1090 w1117 w1154 w1204 w1240 w1320 w1382 w1419 w1477 w1534 w1630 w1708 w1754]
      tunnel: w176 -> [w212 w246 w282 w419 w496 w580 w669 w817 w891 w939 w980 w1022 w1061 w1096 w1124 w1153 w1189 w1275 w1350 w1385 w1443 w1501 w1557 w1641 w1717 w1755]
      tunnel: w175 -> [w211 w245 w281 w418 w495 w579 w668 w816 w890 w938 w979 w1021 w1060 w1095 w1123 w1152 w1190 w1250 w1329 w1384 w1427 w1485 w1542 w1632 w1710 w1757]
      tunnel: [w215 w249 w273 w416 w493 w576 w666 w814 w887 w931 w972 w1016 w1056 w1092 w1119 w1156 w1209 w1241 w1302 w1375 w1420 w1478 w1535 w1583 w1669 w1753] -> w174
      tunnel: [w214 w248 w272 w415 w492 w575 w665 w813 w886 w932 w973 w1017 w1057 w1093 w1120 w1155 w1179 w1251 w1303 w1374 w1428 w1486 w1543 w1582 w1668 w1751] -> w105
      tunnel: [w213 w247 w283 w417 w454 w578 w667 w815 w889 w933 w974 w1014 w1054 w1090 w1117 w1154 w1204 w1240 w1320 w1382 w1419 w1477 w1534 w1630 w1708 w1754] -> w173
      tunnel: [w212 w246 w282 w419 w496 w580 w669 w817 w891 w939 w980 w1022 w1061 w1096 w1124 w1153 w1189 w1275 w1350 w1385 w1443 w1501 w1557 w1641 w1717 w1755] -> w172
      tunnel: [w211 w245 w281 w418 w495 w579 w668 w816 w890 w938 w979 w1021 w1060 w1095 w1123 w1152 w1190 w1250 w1329 w1384 w1427 w1485 w1542 w1632 w1710 w1757] -> w171
      tunnel: [w216 w250 w284 w421 w498 w582 w671 w819 w893 w930 w971 w1015 w1055 w1091 w1118 w1151 w1207 w1249 w1328 w1373 w1426 w1484 w1541 w1631 w1709 w1749] -> w57
      tunnel: w170 -> [_ _ _ w423 w502 w587 w674 w821 w897 _ _ _ _ _ _ _ _ w1246 w1325 _ w1425 w1483 w1540 w1603 w1685 _]
      tunnel: "Gate" -> [_ _ _ w401 w486 w561 w651 w799 w872 _ _ _ _ _ _ _ _ _ _ _ _ _ _ _ _ _]
      tunnel: "Drain 2" -> [_ _ _ w400 w485 w560 w650 w798 w871 _ _ _ _ _ _ _ _ _ _ _ _ _ _ _ _ _]
      tunnel: "Panel Controls" -> [_ _ _ _ _ w559 w649 w688 w870 _ _ _ _ _ _ _ _ _ _ _ _ _ _ _ _ _]
      tunnel: w166 -> [w210 w244 w280 w385 w476 w544 w635 w783 w856 w937 w978 _ w1053 w1089 w1116 w1150 w1191 w1236 w1316 w1378 w1415 w1473 w1530 w1626 w1704 w1758]
      tunnel: w165 -> [w209 w243 w279 w384 w475 w543 w634 w782 w855 w936 w977 w1020 _ w1080 w1122 w1149 w1192 w1237 w1317 w1379 w1416 w1474 w1531 w1627 w1705 w1759]
      tunnel: w164 -> [w208 w242 w278 w383 w474 w542 w633 w781 w854 w935 w976 w1019 w1059 w1094 _ w1148 w1193 w1238 w1318 w1380 w1417 w1475 w1532 w1628 w1706 w1760]
      tunnel: w163 -> [w207 w241 w277 w382 w473 w541 w636 w780 w857 w934 w975 w1018 w1058 _ w1121 w1147 w1194 w1239 w1319 w1381 w1418 w1476 w1533 w1629 w1707 w1761]
      tunnel: [w210 w244 w280 w385 w476 w544 w635 w783 w856 w937 w978 w1013 w1053 w1089 w1116 w1150 w1191 w1236 w1316 w1378 w1415 w1473 w1530 w1626 w1704 w1758] -> w162
      tunnel: [w209 w243 w279 w384 w475 w543 w634 w782 w855 w936 w977 w1020 w1045 w1080 w1122 w1149 w1192 w1237 w1317 w1379 w1416 w1474 w1531 w1627 w1705 w1759] -> w161
      tunnel: [w208 w242 w278 w383 w474 w542 w633 w781 w854 w935 w976 w1019 w1059 w1094 w1115 w1148 w1193 w1238 w1318 w1380 w1417 w1475 w1532 w1628 w1706 w1760] -> w160
      tunnel: [w207 w241 w277 w382 w473 w541 w636 w780 w857 w934 w975 w1018 w1058 w1081 w1121 w1147 w1194 w1239 w1319 w1381 w1418 w1476 w1533 w1629 w1707 w1761] -> w159
      tunnel: w158 -> [_ _ _ w377 w470 _ w629 w775 _ _ _ _ _ _ _ _ _ _ _ _ _ _ _ _ _ _]
      tunnel: w157 -> [_ _ _ w375 w469 _ _ _ _ _ _ _ _ _ _ _ _ _ _ _ _ _ _ _ _ _]
      tunnel: [w206 w237 w270 w307 w446 w531 w626 w706 w843 w929 w969 w1012 w1044 w1079 w1114 w1146 w1175 w1228 w1285 w1372 w1404 w1466 w1524 w1580 w1662 w1750] -> w69
      tunnel: w156 -> [w206 w237 w270 w372 w446 w531 w626 w771 w843 w929 w969 w1012 w1044 w1079 w1114 w1146 w1175 w1228 w1285 w1372 w1404 w1466 w1524 w1580 w1662 w1750]
      tunnel: w123 -> [_ _ _ w369 w443 w529 w624 w768 w840 _ _ _ _ _ _ _ w1173 w1226 w1298 _ w1401 w1463 w1521 w1577 w1658 _]
      tunnel: w154 -> [_ _ _ w366 w442 w527 w623 w765 w839 _ _ _ _ _ _ _ w1171 w1224 w1297 _ w1400 w1462 w1520 w1576 w1659 _]
      tunnel: w106 -> [_ _ _ w361 _ _ _ w760 _ _ _ _ _ _ _ _ _ _ _ _ _ _ _ _ _ _]
      tunnel: [w205 w236 w269 w315 w445 w530 w625 w714 w842 w928 w968 w1011 w1043 w1078 w1113 w1145 w1174 w1227 w1300 w1371 w1403 w1465 w1523 w1579 w1661 w1756] -> w107
      tunnel: w152 -> [w205 w236 w269 w365 w445 w530 w625 w764 w842 w928 w968 w1011 w1043 w1078 w1113 w1145 w1174 w1227 w1300 w1371 w1403 w1465 w1523 w1579 w1661 w1756]
      tunnel: [w204 w235 w268 w306 w441 w526 w622 w705 w838 w927 w967 w1010 w1042 w1077 w1112 w1144 w1170 w1223 w1284 w1370 w1399 w1461 w1519 w1575 w1657 w1745] -> w68
      tunnel: w128 -> [w204 w235 w268 w359 w441 w526 w622 w758 w838 w927 w967 w1010 w1042 w1077 w1112 w1144 w1170 w1223 w1284 w1370 w1399 w1461 w1519 w1575 w1657 w1745]
      tunnel: [w203 w234 w267 w352 w440 w525 w612 w751 w837 w926 w966 w1009 w1041 w1076 w1111 w1143 w1169 w1222 w1296 w1369 w1398 w1460 w1518 w1574 w1656 w1744] -> w101
      tunnel: w114 -> [w203 w234 w267 w352 w440 w525 w612 w751 w837 w926 w966 w1009 w1041 w1076 w1111 w1143 w1169 w1222 w1296 w1369 w1398 w1460 w1518 w1574 w1656 w1743]
      tunnel: [w202 w233 w266 w351 w439 w524 w611 w750 w836 w925 w965 w1008 w1040 w1075 w1110 w1142 w1168 w1221 w1295 w1368 w1397 w1459 w1517 w1573 w1655 w1729] -> w109
      tunnel: w108 -> [w202 w233 w266 w351 w439 w524 w611 w750 w836 w925 w965 w1008 w1040 w1075 w1110 w1142 w1168 w1221 w1295 w1368 w1397 w1459 w1517 w1573 w1655 w1729]
      tunnel: w106 -> [_ _ _ _ _ _ _ _ _ _ _ _ _ _ _ _ _ _ _ _ _ _ _ _ _ _]
      tunnel: [w201 w232 w265 w350 w438 w523 w610 w749 w835 w924 w964 w1007 w1039 w1074 w1109 w1141 w1167 w1220 w1294 w1367 w1396 w1458 w1516 w1572 w1654 w1728] -> w102
      tunnel: w104 -> [w201 w232 w265 w350 w438 w523 w610 w749 w835 w924 w964 w1007 w1039 w1074 w1109 w1141 w1167 w1220 w1294 w1367 w1396 w1458 w1516 w1572 w1654 w1728]
      tunnel: [w199 w230 w263 w300 w435 w521 w608 w699 w833 w922 w963 w1006 w1037 w1072 w1107 w1139 w1165 w1219 w1293 w1366 w1395 w1457 w1514 w1571 w1653 w1727] -> w62
      tunnel: w90 -> [w199 w230 w263 w346 w435 w521 w608 w745 w833 w922 w963 w1006 w1037 w1072 w1107 w1139 w1165 w1219 w1293 w1366 w1395 w1457 w1514 w1571 w1653 w1727]
      tunnel: [w200 w231 w264 w301 w436 w522 w609 w700 w834 w923 w962 w1005 w1038 w1073 w1108 w1140 w1166 w1218 w1292 w1365 w1394 w1456 w1515 w1570 w1652 w1726] -> w63
      tunnel: w89 -> [w200 w231 w264 w345 w436 w522 w609 w744 w834 w923 w962 w1005 w1038 w1073 w1108 w1140 w1166 w1218 w1292 w1365 w1394 w1456 w1515 w1570 w1652 w1726]
      tunnel: [w192 w223 w256 w305 w432 w519 w606 w704 w831 w915 w960 w1003 w1035 w1070 w1105 w1137 w1158 w1211 w1283 w1364 w1387 w1449 w1507 w1563 w1647 w1719] -> w67
      tunnel: w78 -> [w192 w223 w256 w335 w432 w519 w606 w734 w831 w915 w960 w1003 w1035 w1070 w1105 w1137 w1158 w1211 w1283 w1364 w1387 w1449 w1507 w1563 w1647 w1719]
      tunnel: [w191 w222 w255 w304 w433 w520 w607 w703 w832 w914 w961 w1004 w1036 w1071 w1106 w1138 w1157 w1210 w1282 w1363 w1386 w1448 w1506 w1562 w1646 w1718] -> w66
      tunnel: w77 -> [w191 w222 w255 w334 w433 w520 w607 w733 w832 w914 w961 w1004 w1036 w1071 w1106 w1138 w1157 w1210 w1282 w1363 w1386 w1448 w1506 w1562 w1646 w1718]
      tunnel: [w194 w225 w258 w310 w431 w517 w604 w709 w829 w920 w958 w1001 w1033 w1068 w1103 w1135 w1160 w1213 w1287 w1358 w1389 w1451 w1509 w1565 w1645 w1723] -> w60
      tunnel: w76 -> [w194 w225 w258 w331 w431 w517 w604 w730 w829 w920 w958 w1001 w1033 w1068 w1103 w1135 w1160 w1213 w1287 w1358 w1389 w1451 w1509 w1565 w1645 w1723]
      tunnel: [w193 w224 w257 w308 w434 w518 w605 w707 w830 w921 w959 w1002 w1034 w1069 w1104 w1136 w1159 w1212 w1286 w1357 w1388 w1450 w1508 w1564 w1644 w1722] -> w70
      tunnel: w75 -> [w193 w224 w257 w330 w434 w518 w605 w729 w830 w921 w959 w1002 w1034 w1069 w1104 w1136 w1159 w1212 w1286 w1357 w1388 w1450 w1508 w1564 w1644 w1722]
      tunnel: [w196 w227 w260 w299 w430 w515 w602 w698 w827 w918 w956 w999 w1031 w1066 w1101 w1133 w1162 w1215 w1289 w1360 w1391 w1453 w1511 w1567 w1649 w1725] -> w61
      tunnel: w74 -> [w196 w227 w260 w327 w430 w515 w602 w726 w827 w918 w956 w999 w1031 w1066 w1101 w1133 w1162 w1215 w1289 w1360 w1391 w1453 w1511 w1567 w1649 w1725]
      tunnel: [w195 w226 w259 w298 w429 w516 w603 w697 w828 w919 w957 w1000 w1032 w1067 w1102 w1134 w1161 w1214 w1288 w1359 w1390 w1452 w1510 w1566 w1648 w1724] -> w59
      tunnel: w73 -> [w195 w226 w259 w326 w429 w516 w603 w725 w828 w919 w957 w1000 w1032 w1067 w1102 w1134 w1161 w1214 w1288 w1359 w1390 w1452 w1510 w1566 w1648 w1724]
      tunnel: [w198 w229 w262 w303 w428 w513 w600 w702 w825 w916 w954 w997 w1029 w1064 w1099 w1131 w1164 w1217 w1291 w1362 w1393 w1455 w1513 w1569 w1651 w1721] -> w65
      tunnel: w72 -> [w198 w229 w262 w323 w428 w513 w600 w722 w825 w916 w954 w997 w1029 w1064 w1099 w1131 w1164 w1217 w1291 w1362 w1393 w1455 w1513 w1569 w1651 w1721]
      tunnel: [w197 w228 w261 w302 w427 w514 w601 w701 w826 w917 w955 w998 w1030 w1065 w1100 w1132 w1163 w1216 w1290 w1361 w1392 w1454 w1512 w1568 w1650 w1720] -> w64
      tunnel: w71 -> [w197 w228 w261 w322 w427 w514 w601 w721 w826 w917 w955 w998 w1030 w1065 w1100 w1132 w1163 w1216 w1290 w1361 w1392 w1454 w1512 w1568 w1650 w1720]
      frame "wait" {
        n32 = Index Array(array=w221, index=0 ("Index")) -> (element=w219:string)
        n33 = Decimal String To Number(string=w219, default (0L)=u32 0) -> (number=w218:u32)  [unwired: 1 in, 1 out]
        n34 = Wait (ms)(milliseconds to wait=w218) -> ()  [unwired: 1 out]
      }
      frame "wait-min" {
        n35 = Index Array(array=w254, index=0 ("Index")) -> (element=w252:string)
        n36 = Decimal String To Number(string=w252, default (0L)=u32 0) -> (number=w240:u32)  [unwired: 1 in, 1 out]
        n37 = Multiply(x=w240, y=u32 60000) -> (x*y=w239:u32)
        n38 = Wait (ms)(milliseconds to wait=w239) -> ()  [unwired: 1 out]
      }
      frame "standby" {
        n39 = Index Array(array=w286, index=0 ("Index")) -> (element=w276:string)
        n40 = case shown="\"off\", Default" w276 {
          tunnel: [":PAGE:SCON:STAN 0" ":PAGE:SCON:STAN 1"] -> w271
          frame "off", Default {
          }
          frame "on" {
          }
        }
        n41 = VISA Write(VISA resource name=w275, write buffer=w271, error in (no error)=w274) -> (VISA resource name out=w273:refnum<visa-resource-name>, error out=w272:errorcluster)  [unwired: 1 out]
      }
      frame "transfer" {
        # "Adjusts graph colors."
        # "Adjusts graph colors."
        # "Is off"
        # "Is on"
        # "Ion will be the middle element of the array. The calculation of the index is done only once, since Is, Id, and Ig have the same dimensions."
        # "Ig off"
        # "Ig on"
        # "Is min"
        # "Is max"
        # "Ig min"
        # "Ig max"
        # "abs(Ig)"
        # "abs(Is)"
        # "Id min"
        # "Id max"
        # "Y1: Is\nY2: Id\nY3: Ig"
        # "abs(Id)"
        # "Adjusts graph colors."
        # "Adjusts graph colors."
        # "Id off"
        # "Id on"
        # "Adjusts graph colors."
        # "Time array"
        n42 = Delete From Array(array=w414, index=0 ("Index")) -> (deleted portion=w412:string, array with subset deleted=w411:string[])  [unwired: 1 in]
        n43 = Bundle By Name(cluster=w375, "Emergency Stop"=w423) -> (w376:T3)
        n44 = Number To Decimal String(number=w369) -> (decimal integer string=w368:string)  [unwired: 1 in]
        n45 = case shown="\"d\", Default" w412 {
          tunnel: [w425 w426] -> w410
          frame "s" {
            w425 = u16 0 items=["Single", "Double"] ("sweep mode")
          }
          frame "d", Default {
            w426 = u16 1 items=["Single", "Double"] ("sweep mode")
          }
        }
        n46 = Fract/Exp String To Number(string=w411) -> (number=w396:dbl[])  [unwired: 3 in, 1 out]
        n47 = Concatenate Strings(w421, "-transfer-" ("Prefix"), w368, w366, ".txt" ("Suffix (transfer)")) -> (w422:string)
        n48 = VISA Write(VISA resource name=w392, write buffer=":PAGE:CHAN:MODE SWE;" ("write buffer (\"\")"), error in (no error)=w391) -> (VISA resource name out=w389:refnum<visa-resource-name>, error out=w390:errorcluster)  [unwired: 1 out]
        n49 = String To Path(string=w422) -> (path=w420:path)
        n50 = Index Array(array=w396, index #1=0 ("Index")) -> (element #1=w409:dbl, element #2=w408:dbl, element #3=w407:dbl)  [unwired: 2 in]
        n51 = Delete From Array(array=w396, length=3 ("Length"), index=0 ("Index")) -> (array with subset deleted=w394:dbl[])  [unwired: 1 out]
        n52 = Build Array (concatenate)(w365, w361) -> (w315:i32[])
        n53 = Bundle By Name(cluster=w401, "Gate Start"=w409, "Gate Stop"=w408, "Gate Step (linear only)"=w407, "Gate Compliance"=w418, "Range mode"=w385, "Range"=w384) -> (w386:T6)
        n54 = control-ref of="Imax vs time"() -> (w344:refnum<vi>)
        n55 = control-ref of="Imin vs time"() -> (w343:refnum<vi>)
        n56 = control-ref of="Ion vs time"() -> (w312:refnum<vi>)
        n57 = control-ref of="Ioff vs time"() -> (w311:refnum<vi>)
        n58 = control-ref of="I vs Vg"() -> (w370:refnum<vi>)
        n59 = Index Array(array=w394, index #1=0 ("Index")) -> (element #1=w404:dbl, element #2=w403:dbl, element #3=w402:dbl)  [unwired: 2 in]
        n60 = call <vilib>:"compatOverwrite.vi"("overwrite (F)"=TRUE) -> ("overwrite?"=w374:T8)
        n61 = Bundle By Name(cluster=w400, "Drain Start"=w404, "Drain Stop"=w403, "Drain Step"=w402, "Drain Compliance"=w419, "Range mode"=w383, "Range"=w382) -> (w387:T7)
        n62 = call "4155C Transfer.vi"("VISA resource name in"=w389, "Gate"=w386, "Drain"=w387, "Timings"=w417, "error in (no error)"=w390, "SMU4"=w377, "sweep mode"=w410, "Panel Controls"=w376) -> ("VG"=w373:dbl[], "Outparams"=w381:T9, "VISA Resource Name out"=w416:refnum<visa-resource-name>, "IS"=w340:dbl[], "ID"=w342:dbl[], "IG"=w339:dbl[], "error out"=w362:errorcluster, "SMU4"=w378:dbl[])  [unwired: 12 in]
        n63 = Unbundle By Name(w381) -> ("V2 Step"=w380:dbl, "V2 Start"=w379:dbl, "Number of points"=w309:i32)
        n64 = Absolute Value(x=w340) -> (abs(x)=w325:dbl[])
        n65 = Absolute Value(x=w342) -> (abs(x)=w341:dbl[])
        n66 = Absolute Value(x=w339) -> (abs(x)=w328:dbl[])
        n67 = Array Size(array=w341) -> (size(s)=w349:i32)
        n68 = Divide(x=w349, y=2) -> (x/y=w292:dbl)
        n69 = Subtract(x=w292, y=1) -> (x-y=w291:dbl)
        n70 = Array Max & Min(array=w325) -> (max value=w332:dbl, min value=w333:dbl)  [unwired: 2 out]
        n71 = Array Max & Min(array=w341) -> (max value=w371:dbl, min value=w338:dbl)  [unwired: 2 out]
        n72 = Array Max & Min(array=w328) -> (max value=w337:dbl, min value=w336:dbl)  [unwired: 2 out]
        n73 = call "4155C Split array.vi"("Number of VAR2 steps"=w309, "Y2 data in"=w342, "X data in"=w373, "Y1 data in"=w340, "Y3 data in"=w339, "error in (no error)"=w362) -> ("Array of clusters"=w364:cluster{"Y data in":dbl[], "X data in":dbl[]}[], "error out"=w297:errorcluster)  [unwired: 1 in]
        n74 = Index Array(array=w325, index=w291) -> (element=w316:dbl)
        n75 = Index Array(array=w325, index=0) -> (element=w317:dbl)
        n76 = Index Array(array=w341, index=w291) -> (element=w318:dbl)
        n77 = Index Array(array=w341, index=0) -> (element=w319:dbl)
        n78 = Index Array(array=w328, index=w291) -> (element=w321:dbl)
        n79 = Index Array(array=w328, index=0) -> (element=w320:dbl)
        n80 = local write "Ig max"(w337) -> ()
        n81 = local write "Ig min"(w336) -> ()
        n82 = local write "Is max"(w332) -> ()
        n83 = local write "Is min"(w333) -> ()
        n84 = local write "Id max"(w371) -> ()
        n85 = local write "Id min"(w338) -> ()
        n86 = local write "I vs Vg"(w364) -> ()
        n87 = Build Array (concatenate)(w331, w332) -> (w310:dbl[])
        n88 = Build Array (concatenate)(w330, w333) -> (w308:dbl[])
        n89 = local write "Is off"(w317) -> ()
        n90 = local write "Is on"(w316) -> ()
        n91 = Build Array (concatenate)(w372, w371) -> (w307:dbl[])
        n92 = Build Array (concatenate)(w359, w338) -> (w306:dbl[])
        n93 = Build Array (concatenate)(w335, w337) -> (w305:dbl[])
        n94 = Build Array (concatenate)(w334, w336) -> (w304:dbl[])
        n95 = Build Array (concatenate)(w323, w316) -> (w303:dbl[])
        n96 = Build Array (concatenate)(w322, w317) -> (w302:dbl[])
        n97 = Build Array (concatenate)(w345, w318) -> (w301:dbl[])
        n98 = Build Array (concatenate)(w346, w319) -> (w300:dbl[])
        n99 = Build Array (concatenate)(w327, w321) -> (w299:dbl[])
        n100 = Build Array (concatenate)(w326, w320) -> (w298:dbl[])
        n101 = local write "Ig off"(w320) -> ()
        n102 = local write "Ig on"(w321) -> ()
        n103 = local write "Id off"(w319) -> ()
        n104 = local write "Id on"(w318) -> ()
        n105 = call "4155C Split array.vi"("Number of VAR2 steps"=w309, "Y2 data in"=w301, "X data in"=w315, "Y1 data in"=w303, "Y3 data in"=w299, "error in (no error)"=w297) -> ("Array of clusters"=w313:cluster{"Y data in":dbl[], "X data in":dbl[]}[], "error out"=w296:errorcluster)  [unwired: 1 in]
        n106 = call "4155C Split array.vi"("Number of VAR2 steps"=w309, "Y2 data in"=w300, "X data in"=w315, "Y1 data in"=w302, "Y3 data in"=w298, "error in (no error)"=w296) -> ("Array of clusters"=w314:cluster{"Y data in":dbl[], "X data in":dbl[]}[], "error out"=w295:errorcluster)  [unwired: 1 in]
        n107 = call "4155C Split array.vi"("Number of VAR2 steps"=w309, "Y2 data in"=w307, "X data in"=w315, "Y1 data in"=w310, "Y3 data in"=w305, "error in (no error)"=w295) -> ("Array of clusters"=w363:cluster{"Y data in":dbl[], "X data in":dbl[]}[], "error out"=w294:errorcluster)  [unwired: 1 in]
        n108 = call "4155C Split array.vi"("Number of VAR2 steps"=w309, "Y2 data in"=w306, "X data in"=w315, "Y1 data in"=w308, "Y3 data in"=w304, "error in (no error)"=w294) -> ("Array of clusters"=w360:cluster{"Y data in":dbl[], "X data in":dbl[]}[], "error out"=w293:errorcluster)  [unwired: 1 in]
        n109 = Open/Create/Replace File(file path (use dialog)=w420, error in=w293, operation (0:open)=w374) -> (refnum out=w357:refnum<file>, error out=w355:errorcluster)  [unwired: 3 in, 1 out]
        n110 = call "4155C Make Big 2d array.vi"("1D Var1"=w373, "1d IS"=w340, "1d ID"=w342, "1d IG"=w339, "1d SMU4"=w378, "SMU4"=w377, "VAR2 START"=w379, "Number of VAR2 steps"=w309, "VAR2 STEP"=w380, "VAR1 Name"="Vg", "Decimal places in header"=i8 1, "VAR2 Name"="Vd") -> ("Header array"=w358:string[], "Data array"=w356:dbl[][])  [unwired: 14 in]
        n111 = local write "Imax vs time"(w363) -> ()
        n112 = local write "Imin vs time"(w360) -> ()
        n113 = local write "Ion vs time"(w313) -> ()
        n114 = local write "Ioff vs time"(w314) -> ()
        n115 = call "4155C Config Chart Colours.vi"("Numeric"=w309, "XY Graph 2"=w344) -> ()  [unwired: 6 in]
        n116 = call "4155C Config Chart Colours.vi"("Numeric"=w309, "XY Graph 2"=w343) -> ()  [unwired: 6 in]
        n117 = call "4155C Config Chart Colours.vi"("Numeric"=w309, "XY Graph 2"=w312) -> ()  [unwired: 6 in]
        n118 = call "4155C Config Chart Colours.vi"("Numeric"=w309, "XY Graph 2"=w311) -> ()  [unwired: 6 in]
        n119 = call "4155C Config Chart Colours.vi"("Numeric"=w309, "XY Graph 2"=w370) -> ()  [unwired: 6 in]
        n120 = call "4155C Write array to file.vi"("Byte Stream File Refnum"=w357, "Header"=w358, "Data Array"=w356, "error in (no error)"=w355) -> ("dup refnum"=w354:refnum<file>, "error out"=w353:errorcluster)  [unwired: 1 in]
        n121 = Close File(refnum=w354, error in=w353) -> (error out=w415:errorcluster)  [unwired: 1 out]
      }
      frame "pulsedstressV" {
        w452 = 0
        n122 = Number To Decimal String(number=w443) -> (decimal integer string=w499:string)  [unwired: 1 in]
        n123 = Delete From Array(array=w437, index=0 ("Index")) -> (deleted portion=w490:string, array with subset deleted=w489:string[])  [unwired: 1 in]
        n124 = Bundle By Name(cluster=w469, "Emergency Stop"=w502) -> (w471:T3)
        n125 = VISA Write(VISA resource name=w483, write buffer=":PAGE:CHAN:MODE SWE;" ("write buffer (\"\")"), error in (no error)=w482) -> (VISA resource name out=w480:refnum<visa-resource-name>, error out=w481:errorcluster)  [unwired: 1 out]
        n126 = Concatenate Strings(w498, "-pulsedstressV-" ("Substring"), w499, w442, ".txt" ("Substring")) -> (w501:string)
        n127 = case shown="\"d\", Default" w490 {
          tunnel: [w511 w512] -> w488
          frame "s" {
            w511 = u16 0 items=["Single", "Double"] ("sweep mode")
          }
          frame "d", Default {
            w512 = u16 1 items=["Single", "Double"] ("sweep mode")
          }
        }
        n128 = Fract/Exp String To Number(string=w489) -> (number=w484:dbl[])  [unwired: 3 in, 1 out]
        n129 = String To Path(string=w501) -> (path=w497:path)
        n130 = Index Array(array=w484, index #1=0 ("Index")) -> (element #1=w461:dbl, element #2=w460:dbl, element #3=w457:dbl, element #4=w456:dbl, element #5=w455:dbl, element #6=w459:dbl)  [unwired: 5 in]
        n131 = Bundle By Name(cluster=w458, "Pulse period"=w456, "Base voltage"=w457, "Pulse width"=w455) -> (w454:T5)
        n132 = Unbundle By Name(w454) -> ("Pulse period"=w462:dbl)
        n133 = Bundle By Name(cluster=w486, "Gate Start"=w460, "Gate Stop"=w461, "Gate Step (linear only)"=0, "Gate Compliance"=w495, "Range mode"=w476, "Range"=w475) -> (w477:T6)
        n134 = call <vilib>:"compatOverwrite.vi"("overwrite (F)"=TRUE) -> ("overwrite?"=w447:T8)
        n135 = Bundle By Name(cluster=w485, "Drain Start"=w459, "Drain Stop"=w452, "Drain Step"=w452, "Drain Compliance"=w496, "Range mode"=w474, "Range"=w473) -> (w478:T7)
        n136 = call "4155C PulsedStressV.vi"("VISA resource name in"=w480, "sweep mode"=w488, "Panel Controls"=w471, "Gate"=w477, "Drain"=w478, "Timings"=w454, "error in (no error)"=w481, "SMU4"=w470) -> ("VISA Resource Name out"=w493:refnum<visa-resource-name>, "ID"=w450:dbl[], "IG"=w448:dbl[], "Outparams"=w472:T9, "error out"=w494:errorcluster)  [unwired: 3 in]
        n137 = Unbundle By Name(w472) -> ("Number of points"=w449:i32)  [unwired: 2 out]
        n138 = for {
          N: w449 -> [_]
          tunnel: [w508] -> w451 mode=indexing
          tunnel: w462 -> [w510]
          i -> [w509]
          n139 = Multiply(x=w510, y=w509) -> (x*y=w508:dbl)
        }
        n140 = Insert Into Array(array=dbl[][] [] ("Input Array"), new element=w451) -> (w463:dbl[][])  [unwired: 2 in]
        n141 = Insert Into Array(array=w463, new element=w450) -> (w468:dbl[][])  [unwired: 2 in]
        n142 = Insert Into Array(array=w468, new element=w448) -> (w467:dbl[][])  [unwired: 2 in]
        n143 = Transpose 2D Array(2D array=w467) -> (transposed array=w466:dbl[][])
        n144 = Open/Create/Replace File(file path (use dialog)=w497, error in=w494, operation (0:open)=w447) -> (refnum out=w505:refnum<file>, error out=w506:errorcluster)  [unwired: 3 in, 1 out]
        n145 = call "4155C Write array to file.vi"("Byte Stream File Refnum"=w505, "Header"=string[] ["Time /s", "Id /A", "Ig /A"], "Data Array"=w466, "error in (no error)"=w506) -> ("dup refnum"=w503:refnum<file>, "error out"=w504:errorcluster)  [unwired: 1 in]
        n146 = Close File(refnum=w503, error in=w504) -> (error out=w492:errorcluster)  [unwired: 1 out]
      }
      frame "transfer-fpp" {
        n147 = Number To Decimal String(number=w529) -> (decimal integer string=w583:string)  [unwired: 1 in]
        n148 = Bundle By Name(cluster=w559, "Emergency Stop"=w587) -> (w595:T2)
        n149 = Delete From Array(array=w574, index=0 ("Index")) -> (deleted portion=w572:string, array with subset deleted=w571:string[])  [unwired: 1 in]
        n150 = Concatenate Strings(w582, "-transferfpp-" ("Substring"), w583, w527, ".txt" ("Substring")) -> (w585:string)
        n151 = VISA Write(VISA resource name=w551, write buffer=":PAGE:CHAN:MODE SWE;" ("write buffer (\"\")"), error in (no error)=w550) -> (VISA resource name out=w548:refnum<visa-resource-name>, error out=w549:errorcluster)  [unwired: 1 out]
        n152 = case shown="\"d\", Default" w572 {
          tunnel: [w596 w597] -> w570
          frame "s" {
            w596 = u16 0 items=["Single", "Double"] ("sweep mode")
          }
          frame "d", Default {
            w597 = u16 1 items=["Single", "Double"] ("sweep mode")
          }
        }
        n153 = Fract/Exp String To Number(string=w571) -> (number=w555:dbl[])  [unwired: 3 in, 1 out]
        n154 = String To Path(string=w585) -> (path=w581:path)
        n155 = Index Array(array=w555, index #1=0 ("Index")) -> (element #1=w569:dbl, element #2=w568:dbl, element #3=w567:dbl)  [unwired: 2 in]
        n156 = Delete From Array(array=w555, length=3 ("Length"), index=0 ("Index")) -> (array with subset deleted=w553:dbl[])  [unwired: 1 out]
        n157 = Bundle By Name(cluster=w561, "Gate Start"=w569, "Gate Stop"=w568, "Gate Step (linear only)"=w567, "Gate Compliance"=w579, "Range mode"=w544, "Range"=w543) -> (w545:T6)
        n158 = Index Array(array=w553, index #1=0 ("Index")) -> (element #1=w564:dbl, element #2=w563:dbl, element #3=w562:dbl)  [unwired: 2 in]
        n159 = call <vilib>:"compatOverwrite.vi"("overwrite (F)"=TRUE) -> ("overwrite?"=w532:T8)
        n160 = Bundle By Name(cluster=w560, "Drain Start"=w564, "Drain Stop"=w563, "Drain Step"=w562, "Drain Compliance"=w580, "Range mode"=w542, "Range"=w541) -> (w546:T7)
        n161 = call "4155C Transfer-FPP.vi"("VISA resource name in"=w548, "Gate"=w545, "Drain"=w546, "Timings"=w578, "error in (no error)"=w549, "sweep mode"=w570, "Panel Controls"=w595) -> ("VG"=w586:dbl[], "Outparams"=w540:T9, "VISA Resource Name out"=w576:refnum<visa-resource-name>, "Vprobe2"=w536:dbl[], "ID"=w535:dbl[], "IG"=w534:dbl[], "Vprobe1"=w533:dbl[], "error out"=w577:errorcluster)  [unwired: 13 in]
        n162 = Unbundle By Name(w540) -> ("V2 Step"=w539:dbl, "V2 Start"=w538:dbl, "Number of points"=w537:i32)
        n163 = Open/Create/Replace File(file path (use dialog)=w581, error in=w577, operation (0:open)=w532) -> (refnum out=w592:refnum<file>, error out=w593:errorcluster)  [unwired: 3 in, 1 out]
        n164 = call "4155C Make Big 2d array FPP.vi"("1D Var1"=w586, "1d ID"=w535, "1d Vp2"=w536, "1d IG"=w534, "1d Vp1"=w533, "VAR2 START"=w538, "Number of VAR2 steps"=w537, "VAR2 STEP"=w539, "VAR1 Name"="Vg", "Decimal places in header"=i8 1, "VAR2 Name"="Vd") -> ("Header array"=w588:string[], "Data array"=w589:dbl[][])  [unwired: 15 in]
        n165 = call "4155C Write array to file.vi"("Byte Stream File Refnum"=w592, "Header"=w588, "Data Array"=w589, "error in (no error)"=w593) -> ("dup refnum"=w590:refnum<file>, "error out"=w591:errorcluster)  [unwired: 1 in]
        n166 = Close File(refnum=w590, error in=w591) -> (error out=w575:errorcluster)  [unwired: 1 out]
      }
      frame "output" {
        n167 = Number To Decimal String(number=w624) -> (decimal integer string=w672:string)  [unwired: 1 in]
        n168 = Bundle By Name(cluster=w649, "Emergency Stop"=w674) -> (w684:T2)
        n169 = Delete From Array(array=w664, index=0 ("Index")) -> (deleted portion=w662:string, array with subset deleted=w661:string[])  [unwired: 1 in]
        n170 = Concatenate Strings(w671, "-output-" ("Substring"), w672, w623, ".txt" ("Suffix (output)")) -> (w673:string)
        n171 = VISA Write(VISA resource name=w640, write buffer=":PAGE:CHAN:MODE SWE;" ("write buffer (\"\")"), error in (no error)=w637) -> (VISA resource name out=w639:refnum<visa-resource-name>, error out=w638:errorcluster)  [unwired: 1 out]
        n172 = case shown="\"d\", Default" w662 {
          tunnel: [w685 w686] -> w660
          frame "s" {
            w685 = u16 0 items=["Single", "Double"] ("sweep mode")
          }
          frame "d", Default {
            w686 = u16 1 items=["Single", "Double"] ("sweep mode")
          }
        }
        n173 = Fract/Exp String To Number(string=w661) -> (number=w643:dbl[])  [unwired: 3 in, 1 out]
        n174 = String To Path(string=w673) -> (path=w670:path)
        n175 = Index Array(array=w643, index #1=0 ("Index")) -> (element #1=w659:dbl, element #2=w658:dbl, element #3=w657:dbl)  [unwired: 2 in]
        n176 = Delete From Array(array=w643, length=3 ("Length"), index=0 ("Index")) -> (array with subset deleted=w642:dbl[])  [unwired: 1 out]
        n177 = control-ref of="I vs Vd"() -> (w614:refnum<vi>)
        n178 = Bundle By Name(cluster=w651, "Gate Start"=w659, "Gate Stop"=w658, "Gate Step (linear only)"=w657, "Gate Compliance"=w668, "Range mode"=w635, "Range"=w634) -> (w683:T6)
        n179 = Index Array(array=w642, index #1=0 ("Index")) -> (element #1=w654:dbl, element #2=w653:dbl, element #3=w652:dbl)  [unwired: 2 in]
        n180 = call <vilib>:"compatOverwrite.vi"("overwrite (F)"=TRUE) -> ("overwrite?"=w627:T8)
        n181 = Bundle By Name(cluster=w650, "Drain Start"=w654, "Drain Stop"=w653, "Drain Step"=w652, "Drain Compliance"=w669, "Range mode"=w633, "Range"=w636) -> (w682:T7)
        n182 = call "4155C Output.vi"("VISA resource name in"=w639, "Gate"=w683, "Drain"=w682, "Timings"=w667, "error in (no error)"=w638, "SMU4"=w629, "sweep mode"=w660, "Panel controls"=w684) -> ("VD"=w621:dbl[], "Outparams"=w631:T9, "VISA Resource Name out"=w666:refnum<visa-resource-name>, "IS"=w620:dbl[], "ID"=w619:dbl[], "IG"=w618:dbl[], "error out"=w616:errorcluster, "SMU4"=w628:dbl[])  [unwired: 12 in]
        n183 = Unbundle By Name(w631) -> ("V2 Step"=w632:dbl, "V2 Start"=w630:dbl, "Number of points"=w613:i32)
        n184 = call "4155C Split array.vi"("Number of VAR2 steps"=w613, "Y2 data in"=w619, "X data in"=w621, "Y1 data in"=w620, "Y3 data in"=w618, "error in (no error)"=w616) -> ("Array of clusters"=w617:cluster{"Y data in":dbl[], "X data in":dbl[]}[], "error out"=w615:errorcluster)  [unwired: 1 in]
        n185 = local write "I vs Vd"(w617) -> ()
        n186 = call "4155C Config Chart Colours.vi"("Numeric"=w613, "XY Graph 2"=w614) -> ()  [unwired: 6 in]
        n187 = Open/Create/Replace File(file path (use dialog)=w670, error in=w615, operation (0:open)=w627) -> (refnum out=w679:refnum<file>, error out=w680:errorcluster)  [unwired: 3 in, 1 out]
        n188 = call "4155C Make Big 2d array.vi"("1D Var1"=w621, "1d IS"=w620, "1d ID"=w619, "1d IG"=w618, "1d SMU4"=w628, "SMU4"=w629, "VAR2 START"=w630, "Number of VAR2 steps"=w613, "VAR2 STEP"=w632, "VAR1 Name"="Vd", "Decimal places in header"=i8 1, "VAR2 Name"="Vg") -> ("Header array"=w675:string[], "Data array"=w676:dbl[][])  [unwired: 14 in]
        n189 = call "4155C Write array to file.vi"("Byte Stream File Refnum"=w679, "Header"=w675, "Data Array"=w676, "error in (no error)"=w680) -> ("dup refnum"=w677:refnum<file>, "error out"=w678:errorcluster)  [unwired: 1 in]
        n190 = Close File(refnum=w677, error in=w678) -> (error out=w665:errorcluster)  [unwired: 1 out]
      }
      frame "output2" {
        # "Adjusts graph colors."
        # "Adjusts graph colors."
        # "Is off"
        # "Is on"
        # "Ion will be the middle element of the array. The calculation of the index is done only once, since Is, Id, and Ig have the same dimensions."
        # "Ig off"
        # "Ig on"
        # "Is min"
        # "Is max"
        # "Ig min"
        # "Ig max"
        # "abs(Ig)"
        # "abs(Is)"
        # "Id min"
        # "Id max"
        # "Y1: Is\nY2: Id\nY3: Ig"
        # "abs(Id)"
        # "Adjusts graph colors."
        # "Adjusts graph colors."
        # "Id off"
        # "Id on"
        # "Adjusts graph colors."
        # "Time array"
        n191 = Delete From Array(array=w812, index=0 ("Index")) -> (deleted portion=w810:string, array with subset deleted=w809:string[])  [unwired: 1 in]
        n192 = Bundle By Name(cluster=w688, "Emergency Stop"=w821) -> (w774:T2)
        n193 = Number To Decimal String(number=w768) -> (decimal integer string=w767:string)  [unwired: 1 in]
        n194 = case shown="\"d\", Default" w810 {
          tunnel: [w823 w824] -> w808
          frame "s" {
            w823 = u16 0 items=["Single", "Double"] ("sweep mode")
          }
          frame "d", Default {
            w824 = u16 1 items=["Single", "Double"] ("sweep mode")
          }
        }
        n195 = Fract/Exp String To Number(string=w809) -> (number=w794:dbl[])  [unwired: 3 in, 1 out]
        n196 = Concatenate Strings(w819, "-output-" ("Substring"), w767, w765, ".txt" ("Suffix (transfer)")) -> (w820:string)
        n197 = VISA Write(VISA resource name=w790, write buffer=":PAGE:CHAN:MODE SWE;" ("write buffer (\"\")"), error in (no error)=w789) -> (VISA resource name out=w787:refnum<visa-resource-name>, error out=w788:errorcluster)  [unwired: 1 out]
        n198 = String To Path(string=w820) -> (path=w818:path)
        n199 = Index Array(array=w794, index #1=0 ("Index")) -> (element #1=w807:dbl, element #2=w806:dbl, element #3=w805:dbl)  [unwired: 2 in]
        n200 = Delete From Array(array=w794, length=3 ("Length"), index=0 ("Index")) -> (array with subset deleted=w792:dbl[])  [unwired: 1 out]
        n201 = Build Array (concatenate)(w764, w760) -> (w714:i32[])
        n202 = Bundle By Name(cluster=w799, "Gate Start"=w807, "Gate Stop"=w806, "Gate Step (linear only)"=w805, "Gate Compliance"=w816, "Range mode"=w783, "Range"=w782) -> (w784:T6)
        n203 = control-ref of="Imax vs time"() -> (w743:refnum<vi>)
        n204 = control-ref of="Imin vs time"() -> (w742:refnum<vi>)
        n205 = control-ref of="Ion vs time"() -> (w711:refnum<vi>)
        n206 = control-ref of="Ioff vs time"() -> (w710:refnum<vi>)
        n207 = control-ref of="I vs Vg"() -> (w769:refnum<vi>)
        n208 = Index Array(array=w792, index #1=0 ("Index")) -> (element #1=w802:dbl, element #2=w801:dbl, element #3=w800:dbl)  [unwired: 2 in]
        n209 = call <vilib>:"compatOverwrite.vi"("overwrite (F)"=TRUE) -> ("overwrite?"=w773:T8)
        n210 = Bundle By Name(cluster=w798, "Drain Start"=w802, "Drain Stop"=w801, "Drain Step"=w800, "Drain Compliance"=w817, "Range mode"=w781, "Range"=w780) -> (w785:T7)
        n211 = call "4155C Output.vi"("VISA resource name in"=w787, "Gate"=w784, "Drain"=w785, "Timings"=w815, "error in (no error)"=w788, "SMU4"=w775, "sweep mode"=w808, "Panel controls"=w774) -> ("VD"=w772:dbl[], "Outparams"=w779:T9, "VISA Resource Name out"=w814:refnum<visa-resource-name>, "IS"=w739:dbl[], "ID"=w741:dbl[], "IG"=w738:dbl[], "error out"=w761:errorcluster, "SMU4"=w776:dbl[])  [unwired: 12 in]
        n212 = Unbundle By Name(w779) -> ("V2 Step"=w778:dbl, "V2 Start"=w777:dbl, "Number of points"=w708:i32)
        n213 = Absolute Value(x=w739) -> (abs(x)=w724:dbl[])
        n214 = Absolute Value(x=w741) -> (abs(x)=w740:dbl[])
        n215 = Absolute Value(x=w738) -> (abs(x)=w727:dbl[])
        n216 = Array Size(array=w740) -> (size(s)=w748:i32)
        n217 = Divide(x=w748, y=2) -> (x/y=w691:dbl)
        n218 = Subtract(x=w691, y=1) -> (x-y=w690:dbl)
        n219 = Array Max & Min(array=w724) -> (max value=w731:dbl, min value=w732:dbl)  [unwired: 2 out]
        n220 = Array Max & Min(array=w740) -> (max value=w770:dbl, min value=w737:dbl)  [unwired: 2 out]
        n221 = Array Max & Min(array=w727) -> (max value=w736:dbl, min value=w735:dbl)  [unwired: 2 out]
        n222 = call "4155C Split array.vi"("Number of VAR2 steps"=w708, "Y2 data in"=w741, "X data in"=w772, "Y1 data in"=w739, "Y3 data in"=w738, "error in (no error)"=w761) -> ("Array of clusters"=w763:cluster{"Y data in":dbl[], "X data in":dbl[]}[], "error out"=w696:errorcluster)  [unwired: 1 in]
        n223 = Index Array(array=w724, index=w690) -> (element=w715:dbl)
        n224 = Index Array(array=w724, index=0) -> (element=w716:dbl)
        n225 = Index Array(array=w740, index=w690) -> (element=w717:dbl)
        n226 = Index Array(array=w740, index=0) -> (element=w718:dbl)
        n227 = Index Array(array=w727, index=w690) -> (element=w720:dbl)
        n228 = Index Array(array=w727, index=0) -> (element=w719:dbl)
        n229 = local write "Ig max"(w736) -> ()
        n230 = local write "Ig min"(w735) -> ()
        n231 = local write "Is max"(w731) -> ()
        n232 = local write "Is min"(w732) -> ()
        n233 = local write "Id max"(w770) -> ()
        n234 = local write "Id min"(w737) -> ()
        n235 = local write "I vs Vd"(w763) -> ()
        n236 = Build Array (concatenate)(w730, w731) -> (w709:dbl[])
        n237 = Build Array (concatenate)(w729, w732) -> (w707:dbl[])
        n238 = local write "Is off"(w716) -> ()
        n239 = local write "Is on"(w715) -> ()
        n240 = Build Array (concatenate)(w771, w770) -> (w706:dbl[])
        n241 = Build Array (concatenate)(w758, w737) -> (w705:dbl[])
        n242 = Build Array (concatenate)(w734, w736) -> (w704:dbl[])
        n243 = Build Array (concatenate)(w733, w735) -> (w703:dbl[])
        n244 = Build Array (concatenate)(w722, w715) -> (w702:dbl[])
        n245 = Build Array (concatenate)(w721, w716) -> (w701:dbl[])
        n246 = Build Array (concatenate)(w744, w717) -> (w700:dbl[])
        n247 = Build Array (concatenate)(w745, w718) -> (w699:dbl[])
        n248 = Build Array (concatenate)(w726, w720) -> (w698:dbl[])
        n249 = Build Array (concatenate)(w725, w719) -> (w697:dbl[])
        n250 = local write "Ig off"(w719) -> ()
        n251 = local write "Ig on"(w720) -> ()
        n252 = local write "Id off"(w718) -> ()
        n253 = local write "Id on"(w717) -> ()
        n254 = call "4155C Split array.vi"("Number of VAR2 steps"=w708, "Y2 data in"=w700, "X data in"=w714, "Y1 data in"=w702, "Y3 data in"=w698, "error in (no error)"=w696) -> ("Array of clusters"=w712:cluster{"Y data in":dbl[], "X data in":dbl[]}[], "error out"=w695:errorcluster)  [unwired: 1 in]
        n255 = call "4155C Split array.vi"("Number of VAR2 steps"=w708, "Y2 data in"=w699, "X data in"=w714, "Y1 data in"=w701, "Y3 data in"=w697, "error in (no error)"=w695) -> ("Array of clusters"=w713:cluster{"Y data in":dbl[], "X data in":dbl[]}[], "error out"=w694:errorcluster)  [unwired: 1 in]
        n256 = call "4155C Split array.vi"("Number of VAR2 steps"=w708, "Y2 data in"=w706, "X data in"=w714, "Y1 data in"=w709, "Y3 data in"=w704, "error in (no error)"=w694) -> ("Array of clusters"=w762:cluster{"Y data in":dbl[], "X data in":dbl[]}[], "error out"=w693:errorcluster)  [unwired: 1 in]
        n257 = call "4155C Split array.vi"("Number of VAR2 steps"=w708, "Y2 data in"=w705, "X data in"=w714, "Y1 data in"=w707, "Y3 data in"=w703, "error in (no error)"=w693) -> ("Array of clusters"=w759:cluster{"Y data in":dbl[], "X data in":dbl[]}[], "error out"=w692:errorcluster)  [unwired: 1 in]
        n258 = Open/Create/Replace File(file path (use dialog)=w818, error in=w692, operation (0:open)=w773) -> (refnum out=w756:refnum<file>, error out=w754:errorcluster)  [unwired: 3 in, 1 out]
        n259 = call "4155C Make Big 2d array.vi"("1D Var1"=w772, "1d IS"=w739, "1d ID"=w741, "1d IG"=w738, "1d SMU4"=w776, "SMU4"=w775, "VAR2 START"=w777, "Number of VAR2 steps"=w708, "VAR2 STEP"=w778, "VAR1 Name"="Vd", "Decimal places in header"=i8 1, "VAR2 Name"="Vg") -> ("Header array"=w757:string[], "Data array"=w755:dbl[][])  [unwired: 14 in]
        n260 = local write "Imax vs time"(w762) -> ()
        n261 = local write "Imin vs time"(w759) -> ()
        n262 = local write "Ion vs time"(w712) -> ()
        n263 = local write "Ioff vs time"(w713) -> ()
        n264 = call "4155C Config Chart Colours.vi"("Numeric"=w708, "XY Graph 2"=w743) -> ()  [unwired: 6 in]
        n265 = call "4155C Config Chart Colours.vi"("Numeric"=w708, "XY Graph 2"=w742) -> ()  [unwired: 6 in]
        n266 = call "4155C Config Chart Colours.vi"("Numeric"=w708, "XY Graph 2"=w711) -> ()  [unwired: 6 in]
        n267 = call "4155C Config Chart Colours.vi"("Numeric"=w708, "XY Graph 2"=w710) -> ()  [unwired: 6 in]
        n268 = call "4155C Config Chart Colours.vi"("Numeric"=w708, "XY Graph 2"=w769) -> ()  [unwired: 6 in]
        n269 = call "4155C Write array to file.vi"("Byte Stream File Refnum"=w756, "Header"=w757, "Data Array"=w755, "error in (no error)"=w754) -> ("dup refnum"=w753:refnum<file>, "error out"=w752:errorcluster)  [unwired: 1 in]
        n270 = Close File(refnum=w753, error in=w752) -> (error out=w813:errorcluster)  [unwired: 1 out]
      }
      frame "output-fpp" {
        n271 = Number To Decimal String(number=w840) -> (decimal integer string=w894:string)  [unwired: 1 in]
        n272 = Bundle By Name(cluster=w870, "Emergency Stop"=w897) -> (w907:T2)
        n273 = Delete From Array(array=w885, index=0 ("Index")) -> (deleted portion=w883:string, array with subset deleted=w882:string[])  [unwired: 1 in]
        n274 = VISA Write(VISA resource name=w861, write buffer=":PAGE:CHAN:MODE SWE;" ("write buffer (\"\")"), error in (no error)=w858) -> (VISA resource name out=w860:refnum<visa-resource-name>, error out=w859:errorcluster)  [unwired: 1 out]
        n275 = Concatenate Strings(w893, "-outputfpp-" ("Substring"), w894, w839, ".txt" ("Substring")) -> (w896:string)
        n276 = case shown="\"d\", Default" w883 {
          tunnel: [w908 w909] -> w881
          frame "s" {
            w908 = u16 0 items=["Single", "Double"] ("sweep mode")
          }
          frame "d", Default {
            w909 = u16 1 items=["Single", "Double"] ("sweep mode")
          }
        }
        n277 = Fract/Exp String To Number(string=w882) -> (number=w864:dbl[])  [unwired: 3 in, 1 out]
        n278 = String To Path(string=w896) -> (path=w892:path)
        n279 = Index Array(array=w864, index #1=0 ("Index")) -> (element #1=w880:dbl, element #2=w879:dbl, element #3=w878:dbl)  [unwired: 2 in]
        n280 = Delete From Array(array=w864, length=3 ("Length"), index=0 ("Index")) -> (array with subset deleted=w863:dbl[])  [unwired: 1 out]
        n281 = Bundle By Name(cluster=w872, "Gate Start"=w880, "Gate Stop"=w879, "Gate Step (linear only)"=w878, "Gate Compliance"=w890, "Range mode"=w856, "Range"=w855) -> (w906:T6)
        n282 = Index Array(array=w863, index #1=0 ("Index")) -> (element #1=w875:dbl, element #2=w874:dbl, element #3=w873:dbl)  [unwired: 2 in]
        n283 = call <vilib>:"compatOverwrite.vi"("overwrite (F)"=TRUE) -> ("overwrite?"=w844:T8)
        n284 = Bundle By Name(cluster=w871, "Drain Start"=w875, "Drain Stop"=w874, "Drain Step"=w873, "Drain Compliance"=w891, "Range mode"=w854, "Range"=w857) -> (w905:T7)
        n285 = call "4155C Output-FPP.vi"("VISA resource name in"=w860, "Gate"=w906, "Drain"=w905, "Timings"=w889, "error in (no error)"=w859, "sweep mode"=w881, "Panel controls"=w907) -> ("VD"=w849:dbl[], "Outparams"=w852:T9, "VISA Resource Name out"=w887:refnum<visa-resource-name>, "Vprobe2"=w848:dbl[], "ID"=w847:dbl[], "IG"=w846:dbl[], "Vprobe1"=w845:dbl[], "error out"=w888:errorcluster)  [unwired: 13 in]
        n286 = Unbundle By Name(w852) -> ("V2 Step"=w853:dbl, "V2 Start"=w851:dbl, "Number of points"=w850:i32)
        n287 = Open/Create/Replace File(file path (use dialog)=w892, error in=w888, operation (0:open)=w844) -> (refnum out=w902:refnum<file>, error out=w903:errorcluster)  [unwired: 3 in, 1 out]
        n288 = call "4155C Make Big 2d array FPP.vi"("1D Var1"=w849, "1d ID"=w847, "1d Vp2"=w848, "1d IG"=w846, "1d Vp1"=w845, "VAR2 START"=w851, "Number of VAR2 steps"=w850, "VAR2 STEP"=w853, "VAR1 Name"="Vd", "Decimal places in header"=i8 1, "VAR2 Name"="Vg") -> ("Header array"=w898:string[], "Data array"=w899:dbl[][])  [unwired: 15 in]
        n289 = call "4155C Write array to file.vi"("Byte Stream File Refnum"=w902, "Header"=w898, "Data Array"=w899, "error in (no error)"=w903) -> ("dup refnum"=w900:refnum<file>, "error out"=w901:errorcluster)  [unwired: 1 in]
        n290 = Close File(refnum=w900, error in=w901) -> (error out=w886:errorcluster)  [unwired: 1 out]
      }
      frame "itime" {
        n291 = Delete From Array(array=w912, index=1) -> (deleted portion=w911:string)  [unwired: 1 in, 1 out]
        n292 = Delete From Array(array=w912, index=0 ("Index")) -> (deleted portion=w941:string)  [unwired: 1 in, 1 out]
        n293 = Fract/Exp String To Number(string=w911) -> (number=w910:dbl)  [unwired: 3 in, 1 out]
        n294 = case shown="\"l\"" w941 {
          tunnel: w940 -> [w946 w948 w952]
          tunnel: [w945 w947 w951] -> w933
          tunnel: w910 -> [w943 _ w950]
          frame "s" {
            w944 = u32 0 items=["short  ", "medium  ", "long  "] ("integration time 2")
            n295 = Bundle By Name(cluster=w946, "integration time"=w944, "Short/Long integration time"=w943) -> (w945:T5)
          }
          frame "m", Default {
            w949 = u32 1 items=["short  ", "medium  ", "long  "] ("integration time 2")
            n296 = Bundle By Name(cluster=w948, "integration time"=w949) -> (w947:T5)
          }
          frame "l" {
            w953 = u32 2 items=["short  ", "medium  ", "long  "] ("integration time 2")
            n297 = Bundle By Name(cluster=w952, "integration time"=w953, "Short/Long integration time"=w950) -> (w951:T5)
          }
        }
      }
      frame "pulsed" {
        n298 = Delete From Array(array=w982, index=0 ("Index")) -> (deleted portion=w983:string, array with subset deleted=w970:string[])  [unwired: 1 in]
        n299 = case shown="\"on\", Default" w983 {
          tunnel: w981 -> [w993 w996]
          tunnel: [w992 w995] -> w974
          tunnel: w970 -> [w990 _]
          frame "on", Default {
            w991 = u16 1 items=["Continuous", "Pulsed"] ("sweep method")
            n300 = Fract/Exp String To Number(string=w990) -> (number=w988:dbl[])  [unwired: 3 in, 1 out]
            n301 = Index Array(array=w988, index #1=0 ("Index")) -> (element #1=w987:dbl, element #2=w986:dbl, element #3=w985:dbl)  [unwired: 2 in]
            n302 = Bundle By Name(cluster=w993, "sweep method"=w991, "Pulse period"=w987, "Base voltage"=w986, "Pulse width"=w985) -> (w992:T5)
          }
          frame "off" {
            w994 = u16 0 items=["Continuous", "Pulsed"] ("sweep method")
            n303 = Bundle By Name(cluster=w996, "sweep method"=w994) -> (w995:T5)
          }
        }
      }
      frame "gaterangemode" {
        n304 = Delete From Array(array=w1023, index=0 ("Index")) -> (deleted portion=w1024:string)  [unwired: 1 in, 1 out]
        n305 = case shown="\"f\"" w1024 {
          tunnel: [w1026 w1027 w1028] -> w1013
          frame "a", Default {
            w1026 = u16 0 items=["Auto", "Limited", "Fixed"] ("Gate Range\nmode 2")
          }
          frame "f" {
            w1027 = u16 2 items=["Auto", "Limited", "Fixed"] ("Gate Range\nmode 2")
          }
          frame "l" {
            w1028 = u16 1 items=["Auto", "Limited", "Fixed"] ("Gate Range\nmode 2")
          }
        }
      }
      frame "gaterange" {
        (unwired) u8 11 items=["10fA  ", "100fA  ", "1nA  ", "10nA", "100nA", "1uA", "10uA", "100uA", "1mA", "10mA", "100mA", "1A"] ("Gate Range 2")
        n306 = Delete From Array(array=w1062, index=0 ("Index")) -> (deleted portion=w1052:string)  [unwired: 1 in, 1 out]
        n307 = Scan Value(string=w1052, format string="") -> (value=w1050:dbl)  [unwired: 1 in, 1 out]
        n308 = Logarithm Base 10(1:w1050) -> (0:w1049:dbl)
        n309 = Round To Nearest(number=w1049) -> (nearest integer value=w1048:dbl)
        n310 = Add(x=w1048, y=11.0) -> (x+y=w1046:dbl)
        n311 = To Unsigned Byte Integer(number=w1046) -> (unsigned 8bit integer=w1045:u8)
      }
      frame "drainrange" {
        (unwired) u8 11 items=["10fA  ", "100fA  ", "1nA  ", "10nA", "100nA", "1uA", "10uA", "100uA", "1mA", "10mA", "100mA", "1A"] ("Gate Range 2")
        n312 = Delete From Array(array=w1097, index=0 ("Index")) -> (deleted portion=w1088:string)  [unwired: 1 in, 1 out]
        n313 = Scan Value(string=w1088, format string="") -> (value=w1086:dbl)  [unwired: 1 in, 1 out]
        n314 = Logarithm Base 10(1:w1086) -> (0:w1085:dbl)
        n315 = Round To Nearest(number=w1085) -> (nearest integer value=w1084:dbl)
        n316 = Add(x=w1084, y=11.0) -> (x+y=w1082:dbl)
        n317 = To Unsigned Byte Integer(number=w1082) -> (unsigned 8bit integer=w1081:u8)
      }
      frame "drainrangemode" {
        n318 = Delete From Array(array=w1125, index=0 ("Index")) -> (deleted portion=w1126:string)  [unwired: 1 in, 1 out]
        n319 = case shown="\"f\"" w1126 {
          tunnel: [w1128 w1129 w1130] -> w1115
          frame "a", Default {
            w1128 = u16 0 items=["Auto", "Limited", "Fixed"] ("Gate Range\nmode 2")
          }
          frame "f" {
            w1129 = u16 2 items=["Auto", "Limited", "Fixed"] ("Gate Range\nmode 2")
          }
          frame "l" {
            w1130 = u16 1 items=["Auto", "Limited", "Fixed"] ("Gate Range\nmode 2")
          }
        }
      }
      frame "Error", Default {
      }
      frame "logfile" {
        n320 = Number To Decimal String(number=w1173) -> (decimal integer string=w1208:string)  [unwired: 1 in]
        n321 = Concatenate Strings(w1207, "logfile" ("Substring"), w1208, w1171, ".txt" ("Substring")) -> (w1205:string)
        n322 = String To Path(string=w1205) -> (path=w1178:path)
        n323 = Unbundle(w1204) -> ("integration time"=w1203:u32, "Short/Long integration time"=w1202:dbl, "hold time (sec)"=w1201:dbl, "delay time (sec)"=w1200:dbl, "Step Time (0 disables)"=w1199:dbl, "sweep method"=w1198:u16, "Pulse period"=w1197:dbl, "Base voltage"=w1196:dbl, "Pulse width"=w1195:dbl)
        n324 = Build Array(w1203, w1202, w1201, w1200, w1199, w1198, w1197, w1196, w1195, w1189, w1190, w1191, w1192, w1193, w1194) -> (w1182:dbl[])
        n325 = Insert Into Array(array=dbl[][] [] ("Input Array"), new element=w1182) -> (w1181:dbl[][])  [unwired: 2 in]
        n326 = call <vilib>:"compatOverwrite.vi"("overwrite (F)"=TRUE) -> ("overwrite?"=w1176:T8)
        n327 = Open/Create/Replace File(file path (use dialog)=w1178, error in=w1180, operation (0:open)=w1176) -> (refnum out=w1186:refnum<file>, error out=w1185:errorcluster)  [unwired: 3 in, 1 out]
        n328 = call "4155C Write array to file.vi"("Byte Stream File Refnum"=w1186, "Header"=string[] ["Int Time", "Short/Long Itime", "Hold time", "Delay time", "Step time", "Sweep method", "Pulse period", "Base Voltage", "Pulse width", "Drain compliance", "Gate compliance", "Gate range mode", "Gate range", "S/D range mode", "S/D range"], "Data Array"=w1181, "error in (no error)"=w1185) -> ("dup refnum"=w1188:refnum<file>, "error out"=w1187:errorcluster)  [unwired: 1 in]
        n329 = Close File(refnum=w1188, error in=w1187) -> (error out=w1179:errorcluster)  [unwired: 1 out]
      }
      frame "sample" {
        n330 = Number To Decimal String(number=w1226) -> (decimal integer string=w1274:string)  [unwired: 1 in]
        n331 = Fract/Exp String To Number(string=w1271) -> (number=w1232:dbl[])  [unwired: 3 in, 1 out]
        n332 = Concatenate Strings(w1249, "-sample-" ("Substring"), w1274, w1224, ".txt" ("Substring")) -> (w1272:string)
        n333 = Index Array(array=w1232, index=0 ("Index")) -> (element=w1269:dbl)
        n334 = String To Path(string=w1272) -> (path=w1253:path)
        n335 = Index Array(array=w1232, index=2 ("Index")) -> (element=w1265:dbl)
        n336 = Index Array(array=w1232, index=3 ("Index")) -> (element=w1234:dbl)
        n337 = Index Array(array=w1232, index=4 ("Index")) -> (element=w1231:dbl)
        n338 = call "4155C Config Sampling Measurements.vi"("Sampling interval"=w1231, "Sample time"=w1234, "Display on/off"=TRUE, "Timings"=w1240, "Num Points"=w1265, "error in (no error)"=w1276, "Drain Compliance"=w1275, "Gate Compliance"=w1250, "VISA session"=w1277) -> ("error out"=w1278:errorcluster, "dup VISA resource name"=w1279:refnum<visa-resource-name>)  [unwired: 1 in]
        n339 = Index Array(array=w1232, index=1 ("Index")) -> (element=w1266:dbl)
        n340 = call "4155C Take Sample.vi"("Emergency Stop"=w1246, "error in (no error)"=w1278, "Vd"=w1266, "Vg"=w1269, "VISA resource name in"=w1279) -> ("error out"=w1244:errorcluster, "Id"=w1281:dbl[], "Ig"=w1255:dbl[], "VISA Resource Name out"=w1242:refnum<visa-resource-name>, "Is"=w1280:dbl[], "Time"=w1259:dbl[])  [unwired: 1 in]
        n341 = Insert Into Array(array=dbl[][] [] ("Input Array"), new element=w1259) -> (w1258:dbl[][])  [unwired: 2 in]
        n342 = Insert Into Array(array=w1258, new element=w1255) -> (w1257:dbl[][])  [unwired: 2 in]
        n343 = Insert Into Array(array=w1257, new element=w1281) -> (w1256:dbl[][])  [unwired: 2 in]
        n344 = VISA Write(VISA resource name=w1242, write buffer=":DISP ON" ("write buffer (\"\")"), error in (no error)=w1244) -> (VISA resource name out=w1241:refnum<visa-resource-name>, error out=w1243:errorcluster)  [unwired: 1 out]
        n345 = Insert Into Array(array=w1256, new element=w1280) -> (w1248:dbl[][])  [unwired: 2 in]
        n346 = Transpose 2D Array(2D array=w1248) -> (transposed array=w1247:dbl[][])
        n347 = call <vilib>:"compatOverwrite.vi"("overwrite (F)"=TRUE) -> ("overwrite?"=w1229:T8)
        n348 = Open/Create/Replace File(file path (use dialog)=w1253, error in=w1243, operation (0:open)=w1229) -> (refnum out=w1262:refnum<file>, error out=w1261:errorcluster)  [unwired: 3 in, 1 out]
        n349 = call "4155C Write array to file.vi"("Byte Stream File Refnum"=w1262, "Header"=string[] ["Time /s", "Ig /A", "Id /A", "Is /A"], "Data Array"=w1247, "error in (no error)"=w1261) -> ("dup refnum"=w1264:refnum<file>, "error out"=w1263:errorcluster)  [unwired: 1 in]
        n350 = Close File(refnum=w1264, error in=w1263) -> (error out=w1251:errorcluster)  [unwired: 1 out]
      }
      frame "samplei" {
        n351 = Number To Decimal String(number=w1298) -> (decimal integer string=w1349:string)  [unwired: 1 in]
        n352 = Concatenate Strings(w1328, "-samplei-" ("Substring"), w1349, w1297, ".txt" ("Substring")) -> (w1347:string)
        n353 = Fract/Exp String To Number(string=w1346) -> (number=w1313:dbl[])  [unwired: 3 in, 1 out]
        n354 = String To Path(string=w1347) -> (path=w1331:path)
        n355 = Index Array(array=w1313, index=4 ("Index")) -> (element=w1307:dbl)
        n356 = Index Array(array=w1313, index=3 ("Index")) -> (element=w1308:dbl)
        n357 = Index Array(array=w1313, index=1 ("Index")) -> (element=w1310:dbl)
        n358 = Index Array(array=w1313, index=0 ("Index")) -> (element=w1311:dbl)
        n359 = Index Array(array=w1313, index=2 ("Index")) -> (element=w1309:dbl)
        n360 = call "4155C Config SamplingI Measurements.vi"("Sample time"=w1309, "Display on/off"=TRUE, "Timings"=w1320, "Num Points"=w1310, "error in (no error)"=w1351, "Sampling interval"=w1308, "VISA session"=w1352) -> ("error out"=w1353:errorcluster, "dup VISA resource name"=w1354:refnum<visa-resource-name>)  [unwired: 3 in]
        n361 = call "4155C Take SampleI.vi"("Emergency Stop"=w1325, "error in (no error)"=w1353, "Idg 2"=w1311, "Vdg compliance 2"=w1307, "VISA resource name in"=w1354) -> ("error out"=w1323:errorcluster, "Idg"=w1356:dbl[], "Vdg"=w1333:dbl[], "VISA Resource Name out"=w1321:refnum<visa-resource-name>, "Is"=w1355:dbl[], "Time"=w1337:dbl[])  [unwired: 1 in]
        n362 = Insert Into Array(array=dbl[][] [] ("Input Array"), new element=w1337) -> (w1336:dbl[][])  [unwired: 2 in]
        n363 = Insert Into Array(array=w1336, new element=w1333) -> (w1335:dbl[][])  [unwired: 2 in]
        n364 = Insert Into Array(array=w1335, new element=w1356) -> (w1334:dbl[][])  [unwired: 2 in]
        n365 = VISA Write(VISA resource name=w1321, write buffer=":DISP ON" ("write buffer (\"\")"), error in (no error)=w1323) -> (VISA resource name out=w1306:refnum<visa-resource-name>, error out=w1322:errorcluster)  [unwired: 1 out]
        n366 = Insert Into Array(array=w1334, new element=w1355) -> (w1327:dbl[][])  [unwired: 2 in]
        n367 = call <vilib>:"compatOverwrite.vi"("overwrite (F)"=TRUE) -> ("overwrite?"=w1301:T8)
        n368 = Open/Create/Replace File(file path (use dialog)=w1331, error in=w1322, operation (0:open)=w1301) -> (refnum out=w1340:refnum<file>, error out=w1339:errorcluster)  [unwired: 3 in, 1 out]
        n369 = Transpose 2D Array(2D array=w1327) -> (transposed array=w1326:dbl[][])
        n370 = call "4155C Write array to file.vi"("Byte Stream File Refnum"=w1340, "Header"=string[] ["Time /s", "Vdg /V", "Idg /A", "Is /A"], "Data Array"=w1326, "error in (no error)"=w1339) -> ("dup refnum"=w1342:refnum<file>, "error out"=w1341:errorcluster)  [unwired: 1 in]
        n371 = Close File(refnum=w1342, error in=w1341) -> (error out=w1304:errorcluster)  [unwired: 1 out]
        n372 = VISA Write(VISA resource name=w1306, write buffer=";:PAGE:SCON:STAN OFF;:PAGE:CHAN:VSU2:DIS;" ("write buffer (\"\")"), error in (no error)=w1304) -> (VISA resource name out=w1302:refnum<visa-resource-name>, error out=w1303:errorcluster)  [unwired: 1 out]
      }
      frame "#" {
        n373 = VISA Write(VISA resource name=w1377, write buffer=":DISP ON" ("write buffer (\"\")"), error in (no error)=w1376) -> (VISA resource name out=w1375:refnum<visa-resource-name>, error out=w1374:errorcluster)  [unwired: 1 out]
      }
      frame "stressV" {
        n374 = Number To Decimal String(number=w1401) -> (decimal integer string=w1442:string)  [unwired: 1 in]
        n375 = Concatenate Strings(w1426, "-stressV-" ("Substring"), w1442, w1400, ".txt" ("Substring")) -> (w1440:string)
        n376 = Fract/Exp String To Number(string=w1439) -> (number=w1412:dbl[])  [unwired: 3 in, 1 out]
        n377 = String To Path(string=w1440) -> (path=w1430:path)
        n378 = Index Array(array=w1412, index=3 ("Index")) -> (element=w1409:dbl)
        n379 = Index Array(array=w1412, index=1 ("Index")) -> (element=w1407:dbl)
        n380 = Index Array(array=w1412, index=0 ("Index")) -> (element=w1406:dbl)
        n381 = Index Array(array=w1412, index=4 ("Index")) -> (element=w1411:dbl)
        n382 = Index Array(array=w1412, index=2 ("Index")) -> (element=w1408:dbl)
        n383 = call "4155C Config V Stress.vi"("VISA session"=w1445, "ID compliance"=w1409, "VD"=w1407, "VG"=w1406, "IG compliance"=w1408, "error in (no error)"=w1444, "Display on/off"=TRUE) -> ("dup VISA resource name"=w1447:refnum<visa-resource-name>, "error out"=w1446:errorcluster)
        n384 = call "4155C Apply Stress.vi"("error in (no error)"=w1446, "Duration"=w1411, "Emergency Stop"=w1425, "VISA resource name in"=w1447) -> ("error out"=w1423:errorcluster, "VISA Resource Name out"=w1421:refnum<visa-resource-name>)
        n385 = VISA Write(VISA resource name=w1421, write buffer=":DISP ON" ("write buffer (\"\")"), error in (no error)=w1423) -> (VISA resource name out=w1420:refnum<visa-resource-name>, error out=w1422:errorcluster)  [unwired: 1 out]
        n386 = call <vilib>:"compatOverwrite.vi"("overwrite (F)"=TRUE) -> ("overwrite?"=w1405:T8)
        n387 = Open/Create/Replace File(file path (use dialog)=w1430, error in=w1422, operation (0:open)=w1405) -> (refnum out=w1433:refnum<file>, error out=w1432:errorcluster)  [unwired: 3 in, 1 out]
        n388 = call "4155C Write array to file.vi"("Byte Stream File Refnum"=w1433, "Header"=string[] ["V stress completed successfully", ""], "error in (no error)"=w1432) -> ("dup refnum"=w1435:refnum<file>, "error out"=w1434:errorcluster)  [unwired: 2 in]
        n389 = Close File(refnum=w1435, error in=w1434) -> (error out=w1428:errorcluster)  [unwired: 1 out]
      }
      frame "stressI" {
        n390 = Number To Decimal String(number=w1463) -> (decimal integer string=w1500:string)  [unwired: 1 in]
        n391 = Concatenate Strings(w1484, "-stressI-" ("Substring"), w1500, w1462, ".txt" ("Substring")) -> (w1498:string)
        n392 = Fract/Exp String To Number(string=w1497) -> (number=w1472:dbl[])  [unwired: 3 in, 1 out]
        n393 = Index Array(array=w1472, index=1 ("Index")) -> (element=w1468:dbl)
        n394 = Index Array(array=w1472, index=0 ("Index")) -> (element=w1469:dbl)
        n395 = call "4155C Config I Stress.vi"("VISA session"=w1503, "IDG"=w1469, "VDG compliance"=w1468, "error in (no error)"=w1502, "Display on/off"=TRUE) -> ("dup VISA resource name"=w1505:refnum<visa-resource-name>, "error out"=w1504:errorcluster)
        n396 = Index Array(array=w1472, index=2 ("Index")) -> (element=w1470:dbl)
        n397 = String To Path(string=w1498) -> (path=w1488:path)
        n398 = call "4155C Apply Stress.vi"("error in (no error)"=w1504, "Duration"=w1470, "Emergency Stop"=w1483, "VISA resource name in"=w1505) -> ("error out"=w1481:errorcluster, "VISA Resource Name out"=w1479:refnum<visa-resource-name>)
        n399 = VISA Write(VISA resource name=w1479, write buffer=":DISP ON" ("write buffer (\"\")"), error in (no error)=w1481) -> (VISA resource name out=w1478:refnum<visa-resource-name>, error out=w1480:errorcluster)  [unwired: 1 out]
        n400 = call <vilib>:"compatOverwrite.vi"("overwrite (F)"=TRUE) -> ("overwrite?"=w1467:T8)
        n401 = Open/Create/Replace File(file path (use dialog)=w1488, error in=w1480, operation (0:open)=w1467) -> (refnum out=w1491:refnum<file>, error out=w1490:errorcluster)  [unwired: 3 in, 1 out]
        n402 = call "4155C Write array to file.vi"("Byte Stream File Refnum"=w1491, "Header"=string[] ["I stress completed successfully", ""], "error in (no error)"=w1490) -> ("dup refnum"=w1493:refnum<file>, "error out"=w1492:errorcluster)  [unwired: 2 in]
        n403 = Close File(refnum=w1493, error in=w1492) -> (error out=w1486:errorcluster)  [unwired: 1 out]
      }
      frame "vsu2pulse" {
        n404 = Number To Decimal String(number=w1521) -> (decimal integer string=w1556:string)  [unwired: 1 in]
        n405 = Concatenate Strings(w1541, "-vsu2-" ("Substring"), w1556, w1520, ".txt" ("Substring")) -> (w1554:string)
        n406 = Fract/Exp String To Number(string=w1553) -> (number=w1529:dbl[])  [unwired: 3 in, 1 out]
        n407 = String To Path(string=w1554) -> (path=w1545:path)
        n408 = Index Array(array=w1529, index=1 ("Index")) -> (element=w1528:dbl)
        n409 = Index Array(array=w1529, index=0 ("Index")) -> (element=w1526:dbl)
        n410 = call "4155C Config VSU2 Stress.vi"("error in (no error)"=w1558, "VSU2"=w1526, "Display on/off"=TRUE, "VISA session"=w1559) -> ("error out"=w1560:errorcluster, "dup VISA resource name"=w1561:refnum<visa-resource-name>)
        n411 = call "4155C Apply Stress.vi"("error in (no error)"=w1560, "Duration"=w1528, "Emergency Stop"=w1540, "VISA resource name in"=w1561) -> ("error out"=w1538:errorcluster, "VISA Resource Name out"=w1536:refnum<visa-resource-name>)
        n412 = VISA Write(VISA resource name=w1536, write buffer=":DISP ON" ("write buffer (\"\")"), error in (no error)=w1538) -> (VISA resource name out=w1535:refnum<visa-resource-name>, error out=w1537:errorcluster)  [unwired: 1 out]
        n413 = call <vilib>:"compatOverwrite.vi"("overwrite (F)"=TRUE) -> ("overwrite?"=w1525:T8)
        n414 = Open/Create/Replace File(file path (use dialog)=w1545, error in=w1537, operation (0:open)=w1525) -> (refnum out=w1548:refnum<file>, error out=w1547:errorcluster)  [unwired: 3 in, 1 out]
        n415 = call "4155C Write array to file.vi"("Byte Stream File Refnum"=w1548, "Header"=string[] ["VSU2 pulse completed successfully", ""], "error in (no error)"=w1547) -> ("dup refnum"=w1550:refnum<file>, "error out"=w1549:errorcluster)  [unwired: 2 in]
        n416 = Close File(refnum=w1550, error in=w1549) -> (error out=w1543:errorcluster)  [unwired: 1 out]
      }
      frame "sample-fpp" {
        w1588 = string[] ["Time /s", "Id VgVd /A", "Ig VgVd /A", "Vp1 VgVd /V", "Vp2 VgVd /V"] ("Header")
        w1592 = "%d" ("format string")
        n417 = Number To Decimal String(number=w1577) -> (decimal integer string=w1640:string)  [unwired: 1 in]
        n418 = Fract/Exp String To Number(string=w1637) -> (number=w1625:dbl[])  [unwired: 3 in, 1 out]
        n419 = Concatenate Strings(w1631, "-samplefpp-" ("Substring"), w1640, w1576, ".txt" ("Substring")) -> (w1638:string)
        n420 = String To Path(string=w1638) -> (path=w1600:path)
        n421 = Index Array(array=w1625, index=0 ("Index")) -> (element=w1586:dbl)
        n422 = Index Array(array=w1625, index=1 ("Index")) -> (element=w1585:dbl)
        n423 = Index Array(array=w1625, index=2 ("Index")) -> (element=w1633:dbl)
        n424 = Index Array(array=w1625, index=3 ("Index")) -> (element=w1623:dbl)
        n425 = call "4155C Config Sampling Measurements FPP.vi"("VISA session"=w1643, "Num Points"=w1633, "Vg"=w1586, "Display on/off"=TRUE, "Gate Compliance"=w1632, "Drain Compliance"=w1641, "Standby"="Standby", "error in (no error)"=w1642, "Timings"=w1630, "Vd"=w1585, "Sample time"=w1623) -> ("dup VISA resource name"=w1602:refnum<visa-resource-name>, "error out"=w1601:errorcluster)  [unwired: 3 in]
        n426 = Number To Decimal String(number=w1586) -> (decimal integer string=w1612:string)  [unwired: 1 in]
        n427 = call "4155C Take Sample FPP.vi"("VISA resource name in"=w1602, "error in (no error)"=w1601, "Emergency Stop"=w1603) -> ("Time"=w1607:dbl[], "Vp1"=w1617:dbl[], "VISA Resource Name out"=w1583:refnum<visa-resource-name>, "Ig"=w1605:dbl[], "Id"=w1606:dbl[], "Vp2"=w1615:dbl[], "error out"=w1604:errorcluster)  [unwired: 10 in]
        n428 = Insert Into Array(array=dbl[][] [] ("Input Array"), new element=w1607) -> (w1621:dbl[][])  [unwired: 2 in]
        n429 = Number To Decimal String(number=w1585) -> (decimal integer string=w1610:string)  [unwired: 1 in]
        n430 = Insert Into Array(array=w1621, new element=w1606) -> (w1620:dbl[][])  [unwired: 2 in]
        n431 = Concatenate Strings("(Vg = " ("Substring"), w1612, "V, Vd = " ("Substring"), w1610, "V)" ("Substring")) -> (w1608:string)
        n432 = Insert Into Array(array=w1620, new element=w1605) -> (w1619:dbl[][])  [unwired: 2 in]
        n433 = Insert Into Array(array=w1619, new element=w1617) -> (w1616:dbl[][])  [unwired: 2 in]
        n434 = Insert Into Array(array=w1616, new element=w1615) -> (w1584:dbl[][])  [unwired: 2 in]
        n435 = Transpose 2D Array(2D array=w1584) -> (transposed array=w1614:dbl[][])
        n436 = call <vilib>:"compatOverwrite.vi"("overwrite (F)"=TRUE) -> ("overwrite?"=w1581:T8)
        n437 = Open/Create/Replace File(file path (use dialog)=w1600, error in=w1604, operation (0:open)=w1581) -> (refnum out=w1597:refnum<file>, error out=w1598:errorcluster)  [unwired: 3 in, 1 out]
        n438 = Array To Spreadsheet String(array=w1588, 3:w1592) -> (spreadsheet string=w1594:string)  [unwired: 1 in]
        n439 = Search and Replace String(replace all?=TRUE ("replace all? (F)"), input string=w1594, search string="VgVd", replace string=w1608) -> (result string=w1590:string)  [unwired: 4 in, 3 out]
        n440 = Spreadsheet String To Array(format string=w1592, spreadsheet string=w1590, array type (2D Dbl)=w1588) -> (array=w1589:string[])  [unwired: 1 in]
        n441 = call "4155C Write array to file.vi"("Byte Stream File Refnum"=w1597, "Header"=w1589, "Data Array"=w1614, "error in (no error)"=w1598) -> ("dup refnum"=w1595:refnum<file>, "error out"=w1596:errorcluster)  [unwired: 1 in]
        n442 = Close File(refnum=w1595, error in=w1596) -> (error out=w1582:errorcluster)  [unwired: 1 out]
      }
      frame "resample-fpp" {
        w1672 = string[] ["Time /s", "Id VgVd /A", "Ig VgVd /A", "Vp1 VgVd /V", "Vp2 VgVd /V"] ("Header")
        w1676 = "%d" ("format string")
        n443 = Number To Decimal String(number=w1658) -> (decimal integer string=w1716:string)  [unwired: 1 in]
        n444 = Fract/Exp String To Number(string=w1713) -> (number=w1665:dbl[])  [unwired: 3 in, 1 out]
        n445 = Concatenate Strings(w1709, "-resamplefpp-" ("Substring"), w1716, w1659, ".txt" ("Substring")) -> (w1714:string)
        n446 = String To Path(string=w1714) -> (path=w1684:path)
        n447 = Index Array(array=w1665, index=0 ("Index")) -> (element=w1671:dbl)
        n448 = Index Array(array=w1665, index=1 ("Index")) -> (element=w1670:dbl)
        n449 = Number To Decimal String(number=w1671) -> (decimal integer string=w1694:string)  [unwired: 1 in]
        n450 = call "4155C Take Sample FPP.vi"("VISA resource name in"=w1667, "error in (no error)"=w1666, "Emergency Stop"=w1685) -> ("Time"=w1689:dbl[], "Vp1"=w1699:dbl[], "VISA Resource Name out"=w1669:refnum<visa-resource-name>, "Ig"=w1687:dbl[], "Id"=w1688:dbl[], "Vp2"=w1697:dbl[], "error out"=w1686:errorcluster)  [unwired: 10 in]
        n451 = Insert Into Array(array=dbl[][] [] ("Input Array"), new element=w1689) -> (w1703:dbl[][])  [unwired: 2 in]
        n452 = Number To Decimal String(number=w1670) -> (decimal integer string=w1692:string)  [unwired: 1 in]
        n453 = Insert Into Array(array=w1703, new element=w1688) -> (w1702:dbl[][])  [unwired: 2 in]
        n454 = Concatenate Strings("(Vg = " ("Substring"), w1694, "V, Vd = " ("Substring"), w1692, "V)" ("Substring")) -> (w1690:string)
        n455 = Insert Into Array(array=w1702, new element=w1687) -> (w1701:dbl[][])  [unwired: 2 in]
        n456 = Insert Into Array(array=w1701, new element=w1699) -> (w1698:dbl[][])  [unwired: 2 in]
        n457 = Insert Into Array(array=w1698, new element=w1697) -> (w1664:dbl[][])  [unwired: 2 in]
        n458 = call <vilib>:"compatOverwrite.vi"("overwrite (F)"=TRUE) -> ("overwrite?"=w1663:T8)
        n459 = Open/Create/Replace File(file path (use dialog)=w1684, error in=w1686, operation (0:open)=w1663) -> (refnum out=w1681:refnum<file>, error out=w1682:errorcluster)  [unwired: 3 in, 1 out]
        n460 = Array To Spreadsheet String(array=w1672, 3:w1676) -> (spreadsheet string=w1678:string)  [unwired: 1 in]
        n461 = Transpose 2D Array(2D array=w1664) -> (transposed array=w1696:dbl[][])
        n462 = Search and Replace String(replace all?=TRUE ("replace all? (F)"), input string=w1678, search string="VgVd", replace string=w1690) -> (result string=w1674:string)  [unwired: 4 in, 3 out]
        n463 = Spreadsheet String To Array(format string=w1676, spreadsheet string=w1674, array type (2D Dbl)=w1672) -> (array=w1673:string[])  [unwired: 1 in]
        n464 = call "4155C Write array to file.vi"("Byte Stream File Refnum"=w1681, "Header"=w1673, "Data Array"=w1696, "error in (no error)"=w1682) -> ("dup refnum"=w1679:refnum<file>, "error out"=w1680:errorcluster)  [unwired: 1 in]
        n465 = Close File(refnum=w1679, error in=w1680) -> (error out=w1668:errorcluster)  [unwired: 1 out]
      }
      frame "serial" {
        n466 = local read "Termination char\n(0xA = '\\n' = LF)\n(0xD = '\\r' = CR)"() -> (w1739:u8)
        n467 = local read "Enable Termination\nChar (T)"() -> (w1740:bool)
        n468 = Index Array(array=w1747, index=0 ("Index")) -> (element=w1746:string)
        n469 = local read "parity"() -> (w1730:u16)
        n470 = local read "Delay before read (ms)"() -> (w1741:u32)
        n471 = local read "byte count"() -> (w1738:u32)
        n472 = local read "Timeout (ms)"() -> (w1737:u32)
        n473 = local read "VISA resource name"() -> (w1734:refnum<visa-resource-name>)
        n474 = local read "baud rate"() -> (w1733:u32)
        n475 = local read "Serial End Mode for Reads"() -> (w1732:u16)
        n476 = local read "data bits"() -> (w1731:u16)
        n477 = local read "stop bits"() -> (w1736:u16)
        n478 = local read "flow control"() -> (w1735:u16)
        n479 = call "Serial write and read v0.5.vi"("Delay before read (ms)"=w1741, "Termination char\n(0xA = '\\n' = LF)\n(0xD = '\\r' = CR)"=w1739, "Enable Termination\nChar (T)"=w1740, "parity"=w1730, "stop bits"=w1736, "string to write"=w1746, "flow control"=w1735, "byte count"=w1738, "Serial Settings:Serial End Mode for Reads"=w1732, "Timeout (ms)"=w1737, "error in (no error)"=w1752, "VISA resource name"=w1734, "baud rate"=w1733, "data bits"=w1731) -> ("Serial port output"=w1742:string, "error out"=w1751:errorcluster)
        n480 = Build Array (concatenate)(w1742, w1743) -> (w1744:string[])
      }
    }
    n481 = Build Array(w107, w60, w70, w69, w68, w67, w66, w65, w64, w63, w62, w61, w59) -> (w131:dbl[][])
    n482 = Transpose 2D Array(2D array=w131) -> (transposed array=w130:dbl[][])
    n483 = Concatenate Strings(w57, "-Imax_Imin_Ion_Ioff_vs_time.txt" ("Suffix (Imax,Imin,Ion,Ioff)")) -> (w141:string)
    n484 = Build Array(w92, "Is max (A)" ("VAR2 Name"), "Is min (A)" ("VAR2 Name"), "Id max (A)" ("VAR2 Name"), "Id min (A)" ("VAR2 Name"), "Ig max (A)" ("VAR2 Name"), "Ig min (A)" ("VAR2 Name"), "Is on (A)" ("VAR2 Name"), "Is off (A)" ("VAR2 Name"), "Id on (A)" ("VAR2 Name"), "Id off (A)" ("VAR2 Name"), "Ig on (A)" ("VAR2 Name"), "Ig off (A)" ("VAR2 Name")) -> (w136:string[])
    n485 = Array To Spreadsheet String(array=w130, 3:"%e" ("format string")) -> (spreadsheet string=w134:string)  [unwired: 1 in]
    n486 = Array To Spreadsheet String(array=w136, 3:"" ("format string")) -> (spreadsheet string=w135:string)  [unwired: 1 in]
    n487 = String To Path(string=w141) -> (path=w140:path)
    n488 = Build Array(w135, w134) -> (w133:string[])
    n489 = Write to Text File(file (use dialog)=w140, text=w133, error in=w105) -> (refnum out=w142:refnum<file>, error out=w132:errorcluster)  [unwired: 1 in, 1 out]
    n490 = Close File(refnum=w142, error in=w132) -> (error out=w56:errorcluster)  [unwired: 1 out]
    n491 = Concatenate Strings(w57, "-serial_port_output.txt" ("Suffix (serial port log)")) -> (w111:string)
    n492 = String To Path(string=w111) -> (path=w110:path)
    n493 = Build Array(w92, "Serial port input" ("VAR2 Name"), "Pump status" ("VAR2 Name"), "Serial port output: ") -> (w96:string[])
    n494 = Array To Spreadsheet String(array=w102, 3:"" ("format string")) -> (spreadsheet string=w93:string)  [unwired: 1 in]
    n495 = Array To Spreadsheet String(array=w96, 3:"" ("format string")) -> (spreadsheet string=w94:string)  [unwired: 1 in]
    n496 = Build Array(w94, w93) -> (w95:string[])
    n497 = Array To Spreadsheet String(array=w101, 3:"" ("format string")) -> (spreadsheet string=w116:string)  [unwired: 1 in]
    n498 = Write to Text File(file (use dialog)=w110, text=w95, error in=w56) -> (refnum out=w112:refnum<file>, error out=w113:errorcluster)  [unwired: 1 in, 1 out]
    n499 = Close File(refnum=w112, error in=w113) -> (error out=w54:errorcluster)  [unwired: 1 out]
    n500 = local write "Serial port data"(w116) -> ()
  }
  "error out" <- w17
  "Timings Indicator" <- w5
